vi "MegaAwesome_9_26_12b_JW.vi"() -> ()   [LabVIEW 2011]
uses:
  data/MegaAwesome_States.ctl
  <vilib>/Utility/inputDevices.llb/keyboardAcquire.vi
  <vilib>/Utility/file.llb/Read From Spreadsheet File (string).vi
  <vilib>/Utility/file.llb/Write To Spreadsheet File (string).vi
panel:
  out "Image Center X":i32
  in  "Disable Flag":bool
  out "Index":string
  in  "Slider Min":dbl=5.0
  in  "Slider Max":dbl=5.0
  out "Opj X Axis":string
  out "X Axis Display Type":string
  in  "Index-Sat":dbl=5.0
  in  "Index-Lin":dbl=5.0
  in  "IndexLog-Lin":dbl=5.0
  in  "IndexLog-Sat":dbl=5.0 caption="Num Pts"
  out "Lin Id-Log Used":dbl[](array[numeric])
  out "Lin-Vg Array-Log Used":dbl[](array[numeric])
  in  "New: Comments":string
  out "Save Array":string[][](array[string])
  out "Folder Index":i32 caption="Length"
  out "Sat Id-Used":dbl[](array[numeric])
  out "Sat Vg Array-Used":dbl[](array[numeric])
  out "Vg Array-Log-Used":dbl[](array[numeric])
  out "Sat Id-Log-Used":dbl[](array[numeric])
  out "Lin Id-Used":dbl[](array[numeric])
  out "Lin-Vg Array-Used":dbl[](array[numeric])
  out "Lin Vd":dbl
  out "Recorded Prop":T1
  out "Current State":T2
  in  "Main Tab Control":T3(tab)
  in  "Transfer File":path
  out "Transfer Folder":path
  in  "1) Transport":bool caption="2) Transport"
  in  "Image Analysis":bool caption="1) Image Analysis"
  in  "Transport\nFolder":path caption="Transport Folder"
  out "Transport\nFile":path=path "D:/UserData/Desktop/Jeremy/WFU/Research/Programs/VI mods/Image Not Found.png" caption="Transport File"
  in  "Image Folder":path
  out "Image File":path=path "D:/UserData/Desktop/Jeremy/WFU/Research/Programs/VI mods/Image Not Found.png"
  out "Fabrication Prop":T4
  out "Distances":dbl[](array[numeric])
  in  "Zoom":i16(slide)=-3 scale=-5.0..5.0
  in  "Magnification":u16(ring) items=["5x", "10x", "20x", "50x", "80x"]
  in  "Undo Button":bool
  in  "Remove Button":bool
  in  "Transfer Plots":T5(tab)=enum."Saturation"
  in  "Lin-Trans Slider":dbl(slide) step=1.0 scale=-2.0..2.0 scale format="%#_1p"
  out "Sqrt-Lin":cluster{dbl[], dbl[]}[](graph)
  in  "Sat-Trans Slider":dbl(slide) step=1.0 scale=-2.0..2.0 scale format="%#_1p"
  out "Sqrt-Sat":cluster{dbl[], dbl[]}[](graph)
  out "Raw- Lin":cluster{dbl[], dbl[]}[](graph)
  out "Raw- Sat":cluster{dbl[], dbl[]}[](graph)
  in  "Log Plots":enum32{"Linear", "Saturation", "Transport"}(tab)=enum."Saturation"
  in  "Lin-Log Slider":dbl(slide) step=1.0 scale=-2.0..2.0 scale format="%#_1p"
  out "Lin-Log":cluster{dbl[], dbl[]}[](graph)
  in  "Sat-Log Slider":dbl(slide) step=1.0 scale=-2.0..2.0 scale format="%#_1p"
  out "Sat-Log":cluster{dbl[], dbl[]}[](graph)
  out "Transport":cluster{ext[], ext[]}[](graph)
  out "Transport Name:":string
  in  "Manual Controls":T6
  in  "File Controls":T7
  out "Date Recorded":string="Date Recorded" caption="Measured"
  out "Data Name:":string
  out "Image Name":string
  out "Date Created":string caption="Fabricated"
  in  "Comments:":string
  out "Rec: Length":dbl caption="Length" format="%#_3g"
  out "Rec: Width":dbl caption="Width" format="%#_4g"
  out "Rec: Dielectric (d)":dbl caption="Dielectric (d)" format="%#_3g"
  in  "New: Dielectric":dbl
  in  "New: Length":dbl
  in  "New: Width":dbl
  out "Rec: Temp":dbl caption="Sample Temp" format="%.1f"
  in  "New: Temp":dbl format="%.1f"
  out "Image Out":T8(plugin-control)
  in  "Num Pts":dbl=5.0
  in  "Num Pts Log":dbl=5.0 caption="Num Pts"
  out "Recorded Values Cluster":T9
  out "Calculated Values Cluster":T9 caption="Recorded Values Cluster"
  out "Re-Calculated Values Cluster":T9 caption="Recorded Values Cluster"
  in  "Independant Variable:":string(combo)="Length (um):"
  out "Image Preview":T8(plugin-control)
  out "Total Width":dbl
  in  "Index Array":u16(ring) caption="Index" items=["1A", "1A", "1A", "1A", "1A", "1A", "1A", "1A", "1A", "1A", "1A", "1A", "1A", "1A", "1A", "1A", "1A", "1A", "1A", "1A", "1A", "1A", "1A", "1A", "1A", "1A", "1A", "1A", "1A", "1A", "1A", "1A", "1A", "1A", "1A", "1A", "1A"]
  in  "Room Temp":dbl=294.0 caption="Room Temp (K)"
  out "No Image\n File":path=path "\\\\acad1\\physics/Jurchescu-group/JW-PD/Mega Awesome/Image Not Found.png" caption="No Image File"
  out "Origin Project File":path=path "\\\\acad1\\physics/Jurchescu-group/JW-PD/Group Library/Origin Project Files/DeviceData_8_10_12a_JW.opj"
  out "No Transport\n File":path=path "\\\\acad1\\physics/Jurchescu-group/JW-PD/Mega Awesome/No Transport File.txt" caption="No Transport File"
  in  "Transport Style Controls":T10={"Transport Line Size"=1, "Transport Line Color"=16772608} {"Transport Line Size" items=["Extra Small", "Small", "Medium", "Large", "Extra Large"]}
  out "Application Directory":path
  # "1)  Select the Transfer File that you would like to analyze:"
  # "Transfer Location"
  # "2) What else would you like to view during your analysis?"
  # "Transport Location"
  # "Image Location"
  # "Recorded"
  # "Calculated"
  # "Re-Calculated"
  # "Manual"
  # "um"
  # "Slider\nDoesn't\nWork"
  # "V"
  # "V"
  # "Slider\nDoesn't\nWork"
  # "V"
  # "Default File Choices"
  # "Default Analysis Values"
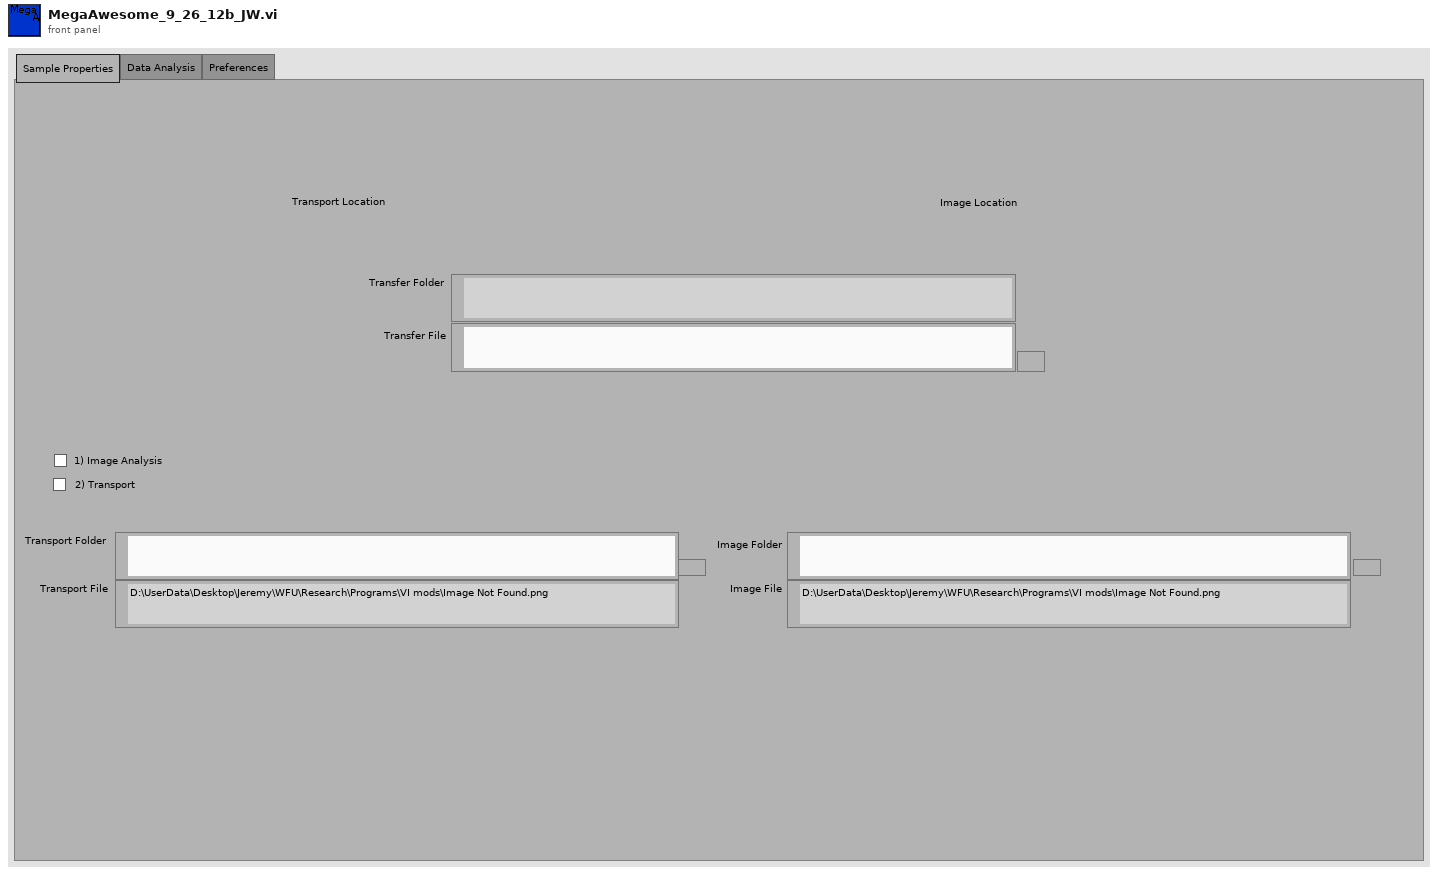
[diagram p1: front panel]
types:
  T1 = cluster{"Date Recorded":string, "Index":string, "Length":dbl, "Width":dbl, "Sample Temp":dbl}
  T2 = typedef "MegaAwesome_States.ctl" = enum16{"Init", "File Missing", "No Event", "Read Data", "Calculated Values", "Re-Calculated Values", "Next File", "Previous File", "Discard File", "Save", "Save Lines", "Export", "Exit"}
  T3 = enum32{"Sample Properties", "Data Analysis", "Preferences"}
  T4 = cluster{"Date Created":string, "Material":string, "Solvent":string, "Concentration":dbl, "Method":string, "Dielectric (nm)":dbl, "Treatment":string, "Comments":string}
  T5 = enum32{"Linear", "Saturation", "Raw-Linear", "Raw-Saturation"}
  T6 = cluster{"Manual-Temp":bool, "Manual-Width":bool, "Manuel-Length":bool, "Manuel-Dielectric":bool, "Manual Comments":bool}
  T7 = cluster{"Previous File":bool, "Discard ":bool, "Save Lines":bool, "Close":bool, "Next File ":bool, "Save":bool, "Save Next":bool, "Export":bool}
  T8 = typedef "IMAQ Image.ctl" = refnum<image>
  T9 = cluster{"Mobility-Sat":dbl, "Moblitity-Lin":dbl, "On/Off":dbl, "Off Current":dbl, "Vt-Sat":dbl, "STS":dbl, "Trap Density-VT":dbl, "Trap Density-STS":dbl}
  T10 = cluster{"Transport Line Size":u16, "Transport Line Color":u32}
  T11 = typedef "LVBoundsTypeDef.ctl" = cluster{"Width":u32, "Height":u32}
  T12 = cluster{"Global Rectangle":i32[], "Contours":cluster{"Contour Type":u32, "ROI Type":u32, "Points":i32[]}[]}
  T13 = cluster{"Contour Type":u32, "ROI Type":u32, "Points":i32[]}[]
  T14 = cluster{i32[], cluster{"Contour Type":u32, "ROI Type":u32, "Points":i32[]}[]}
  T15 = enum16{"0", "1", "2", "3", "4", "5", "6", "7", "8", "9", "A", "B", "C", "D", "E", "F", "G", "H", "I", "J", "K", "L", "M", "N", "O", "P", "Q", "R", "S", "T", "U", "V", "W", "X", "Y", "Z", "F1", "F2", "F3", "F4", "F5", "F6", "F7", "F8", "F9", "F10", "F11", "F12", "F13", "F14", "F15", "ADD", "BACK", "BACKSLASH", "CAPITAL", "COMMA", "DECIMAL", "DELETE", "DIVIDE", "DOWN", "END", "EQUALS", "ESCAPE", "GRAVE (`)", "HOME", "INSERT", "LBRACKET", "LCONTROL", "LEFT", "L ALT", "LSHIFT", "LWIN", "MINUS", "MULTIPLY", "NEXT", "NUMLOCK", "NUMPAD_0", "NUMPAD_1", "NUMPAD_2", "NUMPAD_3", "NUMPAD_4", "NUMPAD_5", "NUMPAD_6", "NUMPAD_7", "NUMPAD_8", "NUMPAD_9", "PAUSE", "PERIOD", "PRIOR (PG UP)", "RBRACKET", "RCONTROL", "RETURN", "RIGHT", "R ALT", "RSHIFT", "RWIN", "SCROLL", "SEMICOLON", "SLASH", "SPACE", "SUBTRACT", "TAB", "UP", "ENTER (num pad)", "' (quote)"}[]
  T16 = enum16{"0", "1", "2", "3", "4", "5", "6", "7", "8", "9", "A", "B", "C", "D", "E", "F", "G", "H", "I", "J", "K", "L", "M", "N", "O", "P", "Q", "R", "S", "T", "U", "V", "W", "X", "Y", "Z", "F1", "F2", "F3", "F4", "F5", "F6", "F7", "F8", "F9", "F10", "F11", "F12", "F13", "F14", "F15", "ADD", "BACK", "BACKSLASH", "CAPITAL", "COMMA", "DECIMAL", "DELETE", "DIVIDE", "DOWN", "END", "EQUALS", "ESCAPE", "GRAVE (`)", "HOME", "INSERT", "LBRACKET", "LCONTROL", "LEFT", "L ALT", "LSHIFT", "LWIN", "MINUS", "MULTIPLY", "NEXT", "NUMLOCK", "NUMPAD_0", "NUMPAD_1", "NUMPAD_2", "NUMPAD_3", "NUMPAD_4", "NUMPAD_5", "NUMPAD_6", "NUMPAD_7", "NUMPAD_8", "NUMPAD_9", "PAUSE", "PERIOD", "PRIOR (PG UP)", "RBRACKET", "RCONTROL", "RETURN", "RIGHT", "R ALT", "RSHIFT", "RWIN", "SCROLL", "SEMICOLON", "SLASH", "SPACE", "SUBTRACT", "TAB", "UP", "ENTER (num pad)", "' (quote)"}
  T17 = typedef "ROI Descriptor" = cluster{"Global Rectangle":i32[], "Contours":cluster{"ID":enum32{"External", "Internal"}, "Type":u32, "Coordinates":i32[]}[]}
  T18 = cluster{string, sgl, bool, bool, bool, bool, bool, bool, i32}
  T19 = cluster{i32, cluster{string, sgl, bool, bool, bool, bool, bool, bool, i32}, i32, i32}
  T20 = cluster{"Contour Type":u32, "ROI Type":u32, "Points":i32[]}
  T21 = cluster{"Points[0]":i32, "Points[1]":i32, "Points[2]":i32, "Points[3]":i32, "Points[4]":i32, "Points[5]":i32, "Points[6]":i32, "Points[7]":i32, "Points[8]":i32}
  T22 = cluster{"[0]":cluster{dbl[], dbl[]}, "[1]":cluster{dbl[], dbl[]}, "[2]":cluster{dbl[], dbl[]}, "[3]":cluster{dbl[], dbl[]}, "[4]":cluster{dbl[], dbl[]}, "[5]":cluster{dbl[], dbl[]}, "[6]":cluster{dbl[], dbl[]}, "[7]":cluster{dbl[], dbl[]}, "[8]":cluster{dbl[], dbl[]}}
  T23 = cluster{"Sat Vg Used":dbl[], "Sat Sqrt(Id) Used ":dbl[], "Lin Vg Used":dbl[], "Lin Sqrt(Id) Used":dbl[], "Index-Lin":dbl, "Index-Sat":dbl}
  T24 = cluster{"Raw Sat":cluster{dbl[], dbl[]}[], "Sqrt Sat":cluster{dbl[], dbl[]}[], "Log Sat":cluster{dbl[], dbl[]}[], "Raw Lin":cluster{dbl[], dbl[]}[], "Sqrt Lin":cluster{dbl[], dbl[]}[], "Log Lin":cluster{dbl[], dbl[]}[]}
  T25 = cluster{"Mobility-Sat":dbl, "Vt-Sat":dbl, "Mobility-Lin":dbl, "Vt-Lin":dbl, "Off I-Sat":dbl, "On/Off I-Sat":dbl}
  T26 = cluster{"Sat Vg Used":dbl[], "Sat Log(Id) Used":dbl[], "Lin Vg Used":dbl[], "Lin Log(Id) Used":dbl[], "STS Index-Sat":dbl, "STS Index-Lin":dbl}
  T27 = cluster{"Independant  Variable Indicator":string, "Parameter String Indicator":string}
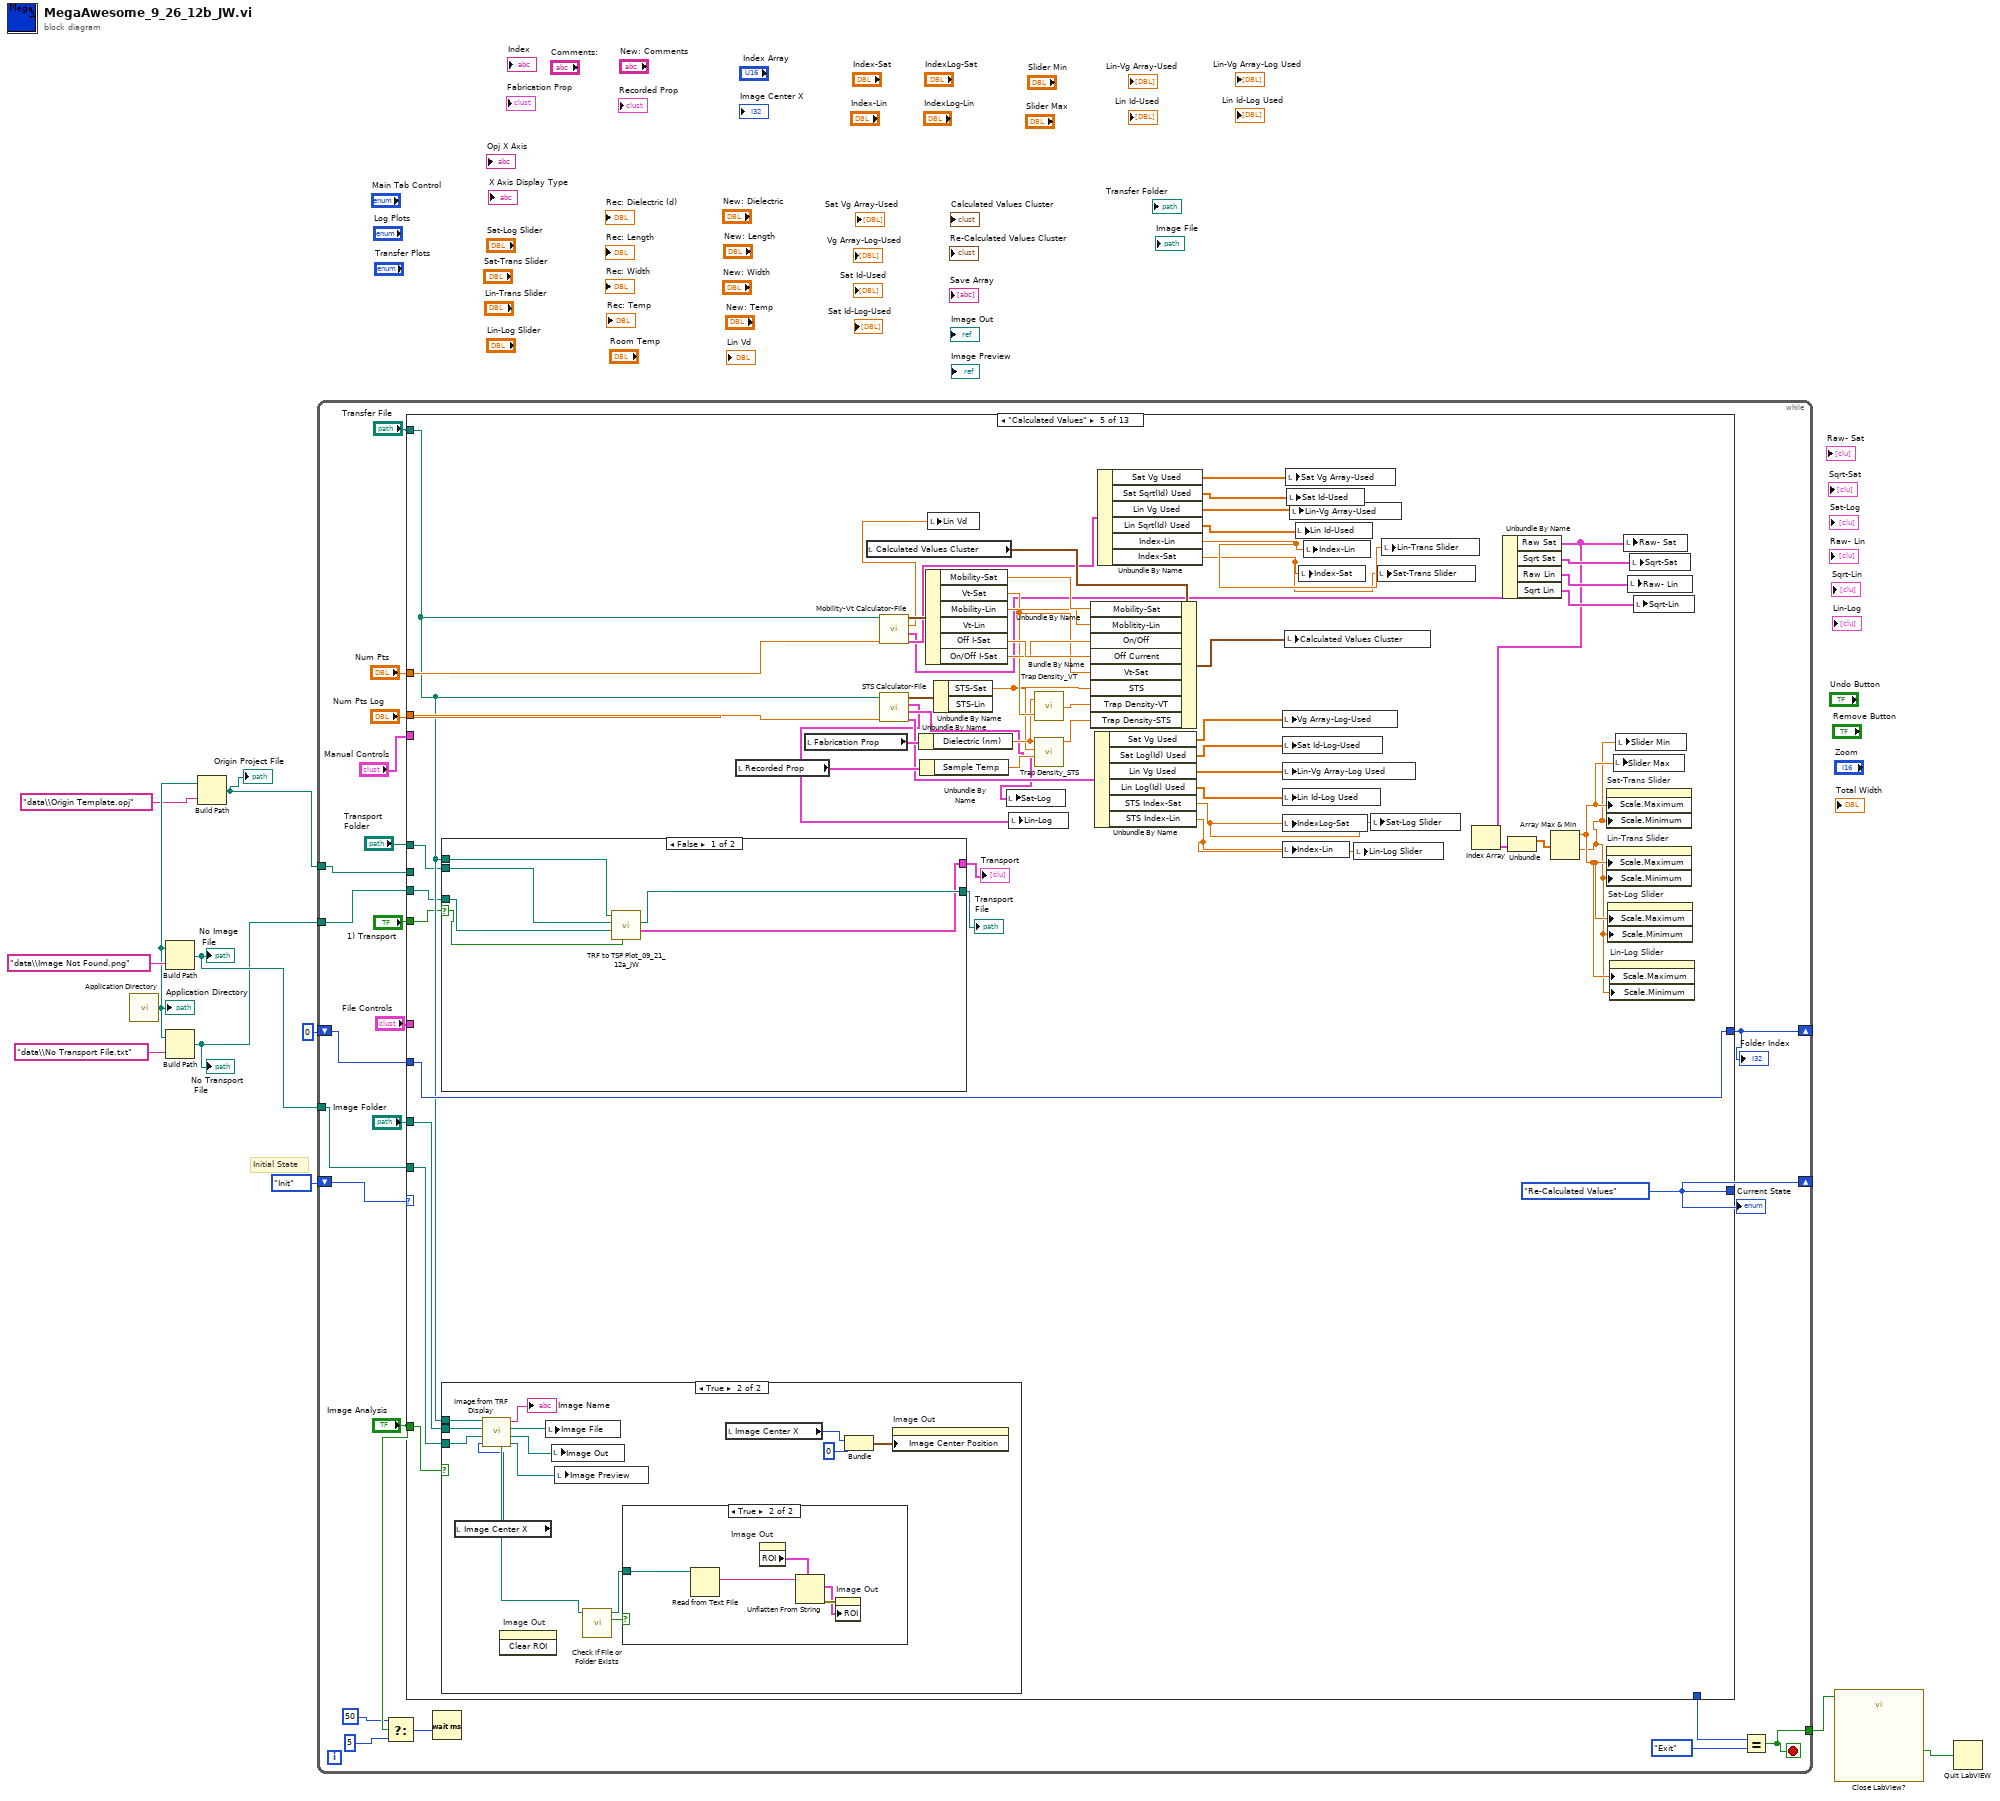
[diagram p0: block diagram]
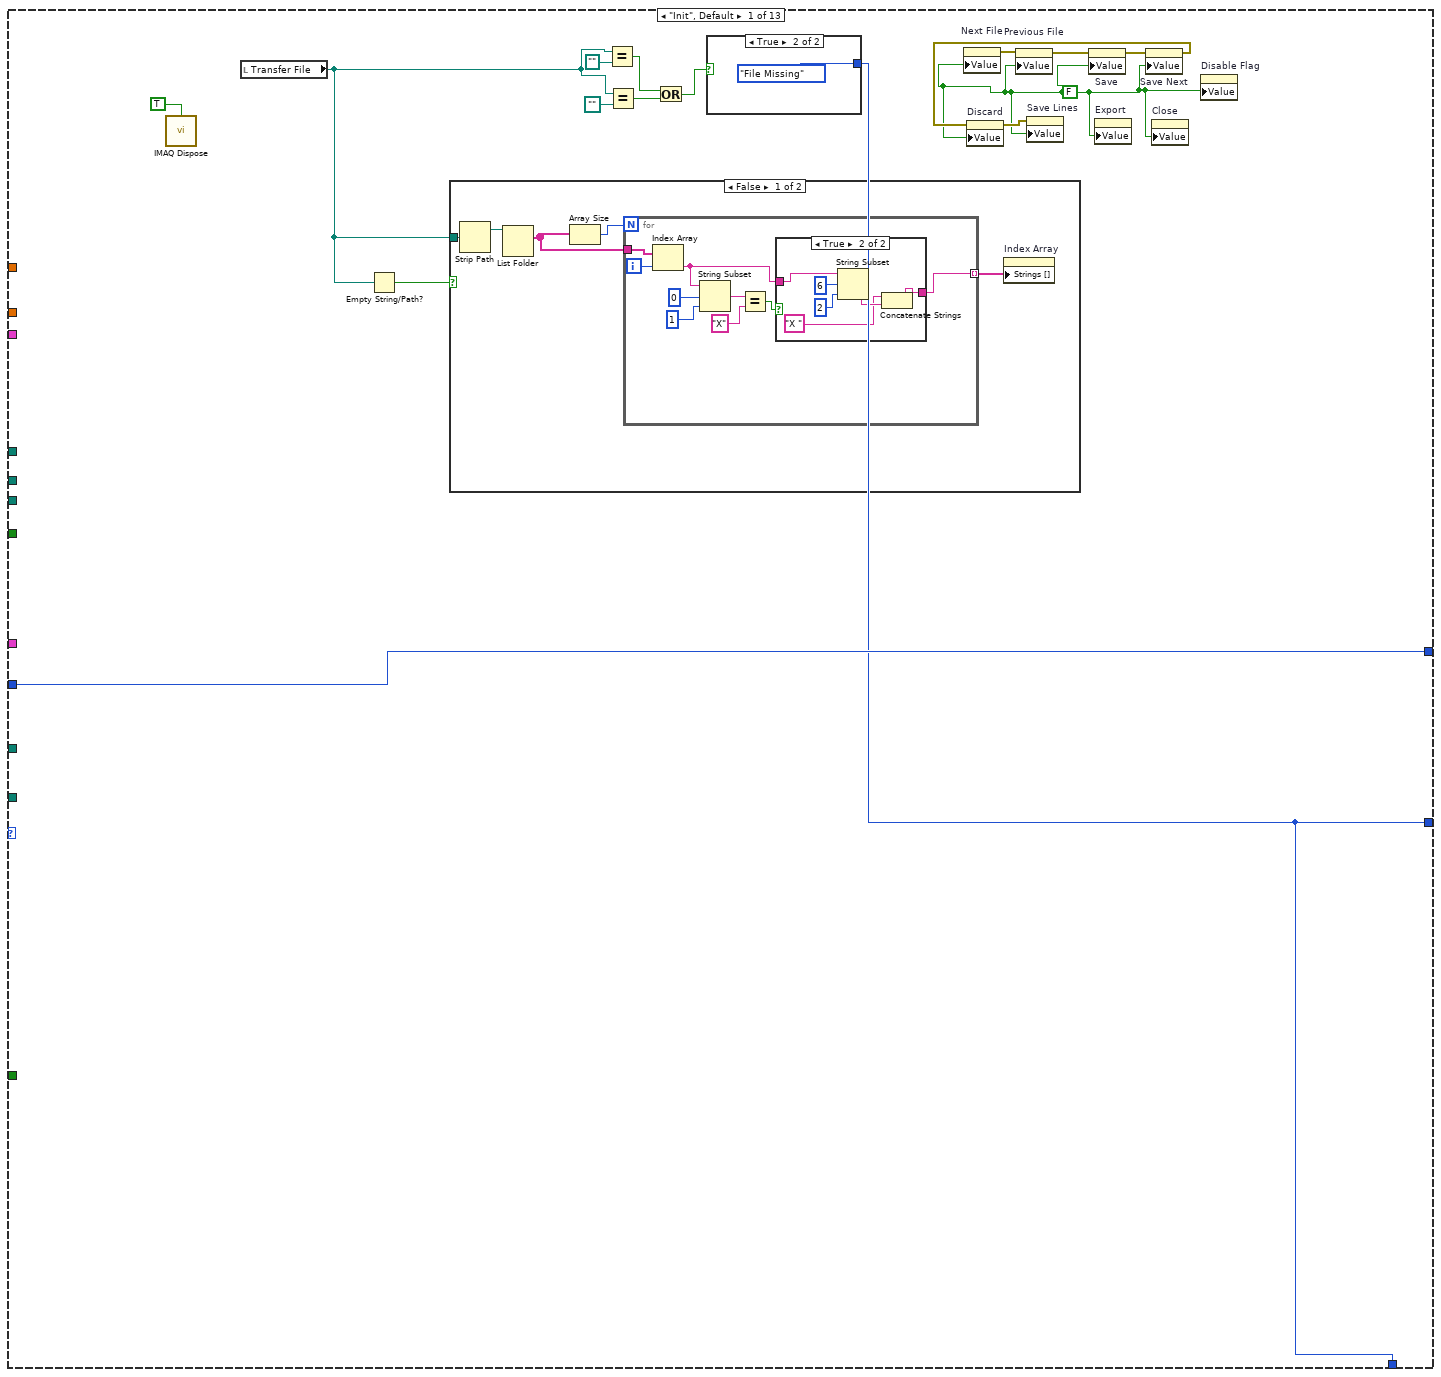
[diagram p2: hidden frame]
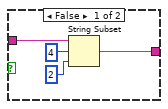
[diagram p3: hidden frame]
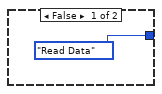
[diagram p5: hidden frame]
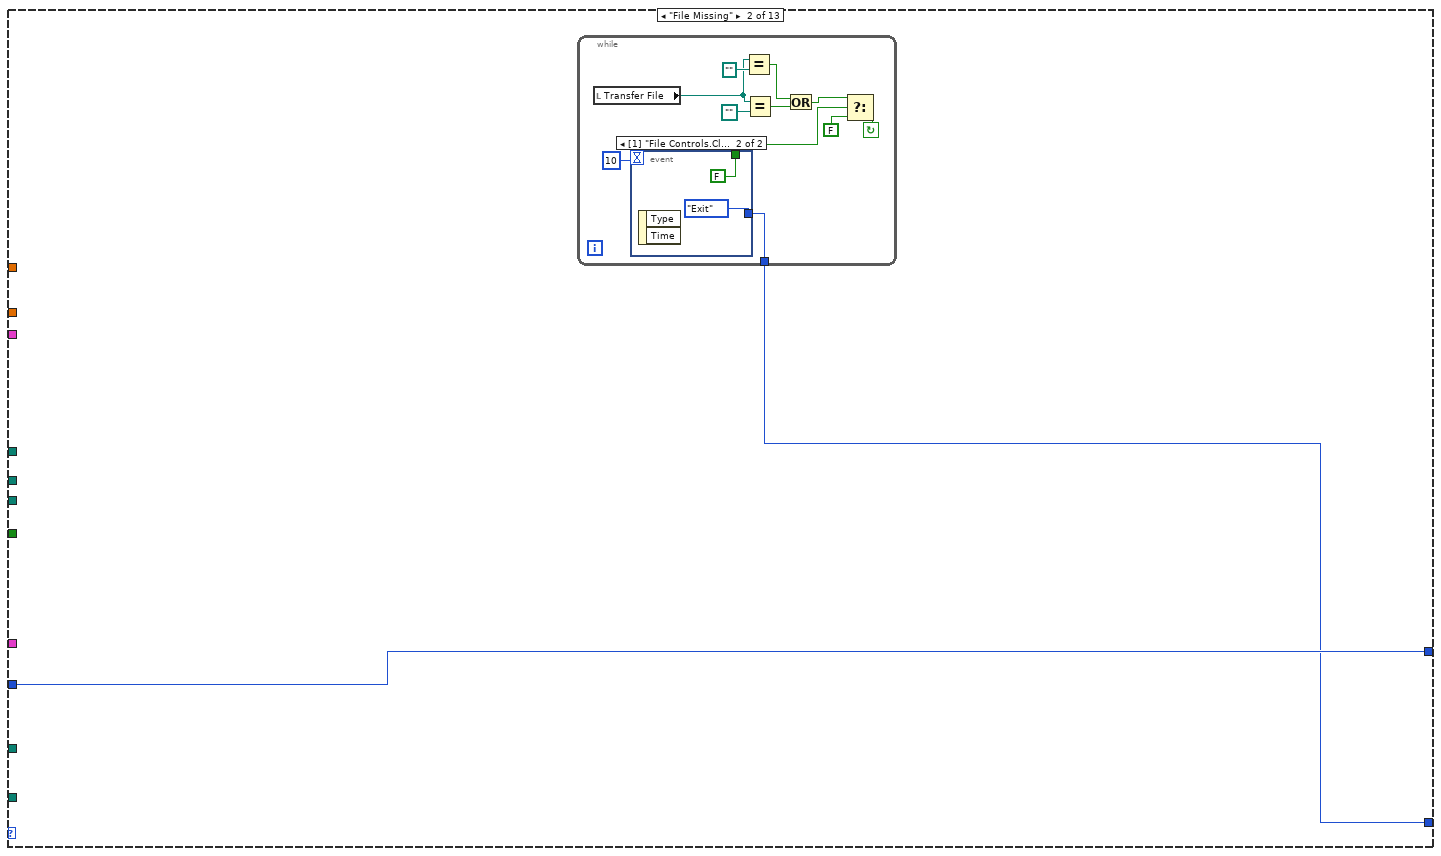
[diagram p6: hidden frame]
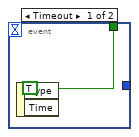
[diagram p7: hidden frame]
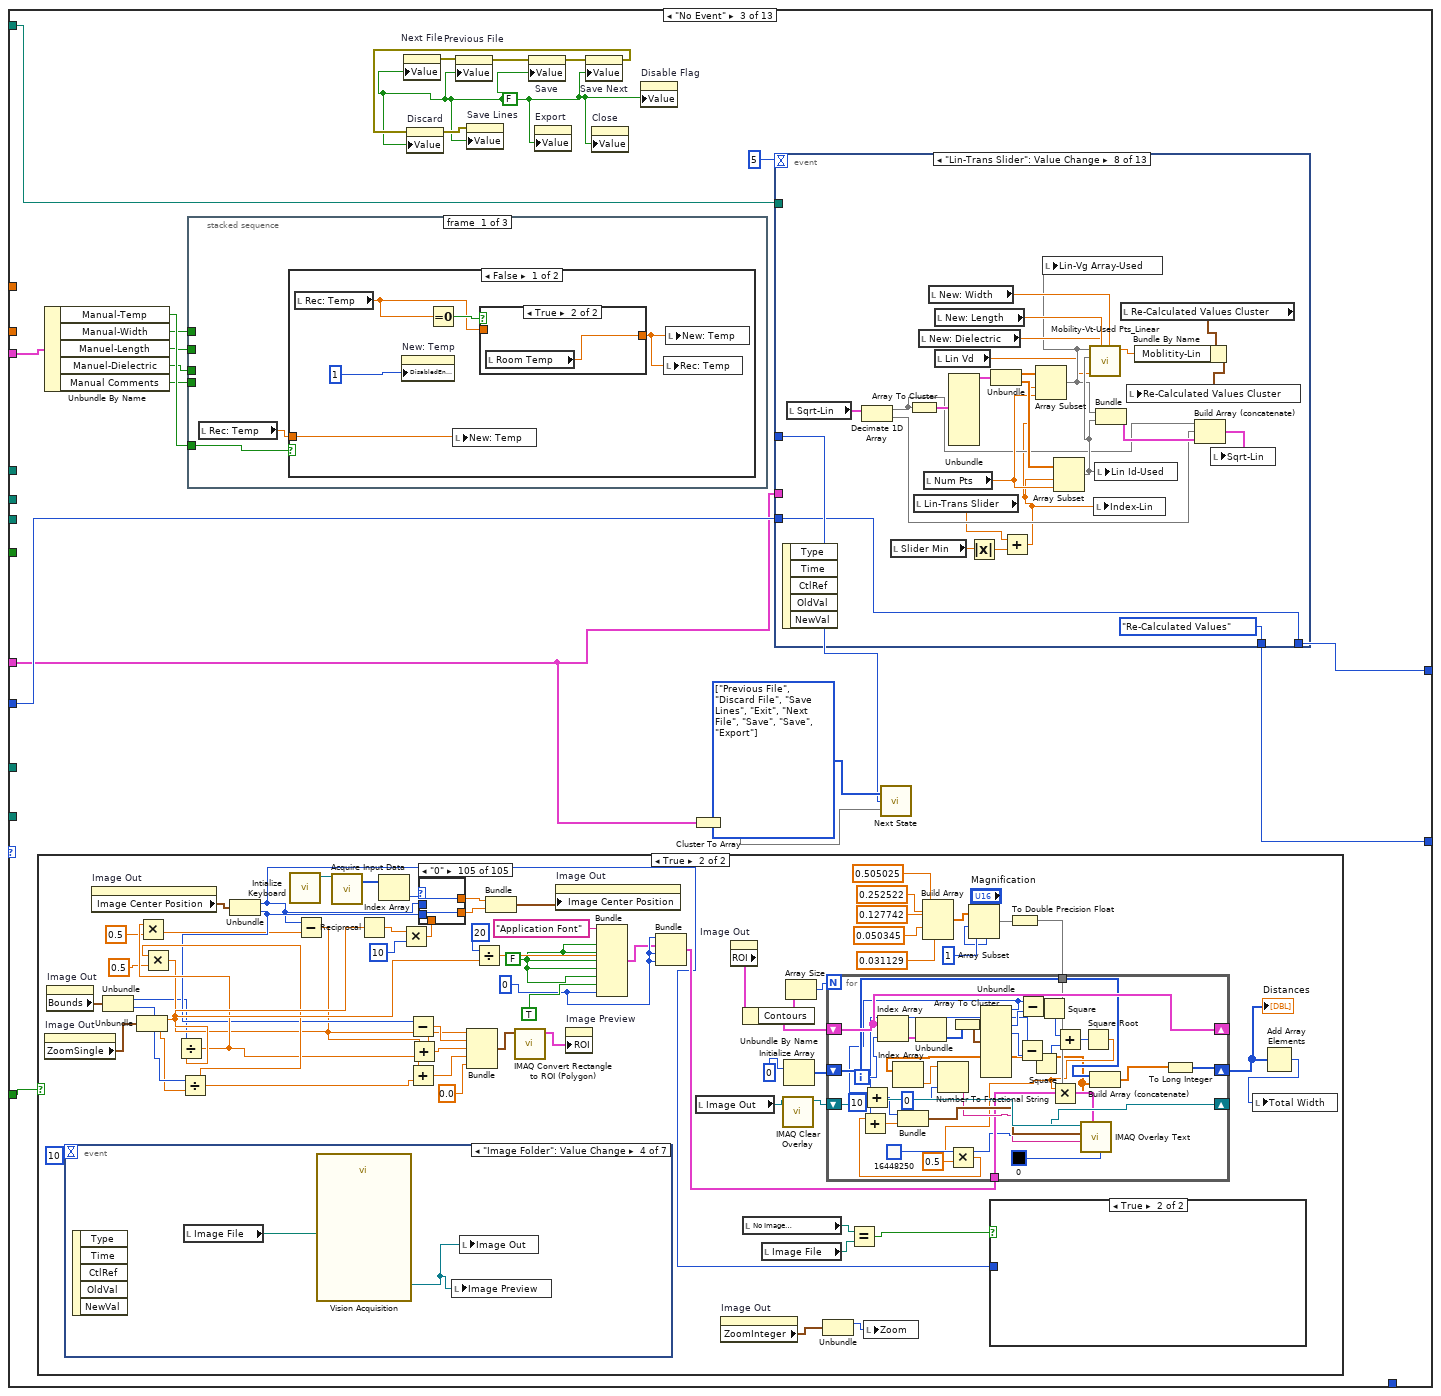
[diagram p8: hidden frame]
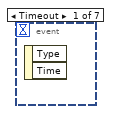
[diagram p10: hidden frame]
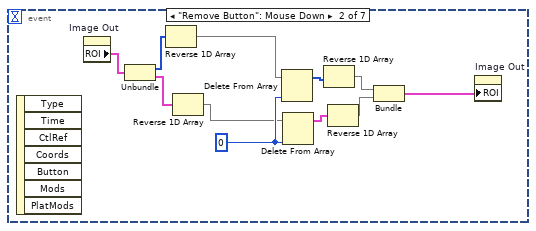
[diagram p11: hidden frame]
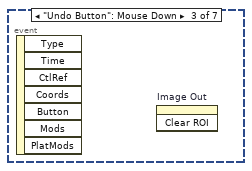
[diagram p12: hidden frame]
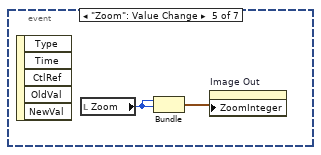
[diagram p13: hidden frame]
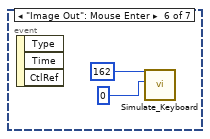
[diagram p14: hidden frame]
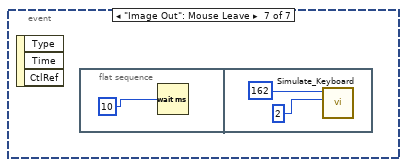
[diagram p15: hidden frame]
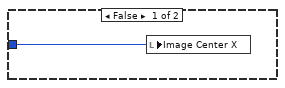
[diagram p16: hidden frame]
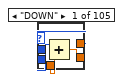
[diagram p17: hidden frame]
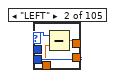
[diagram p18: hidden frame]
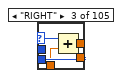
[diagram p19: hidden frame]
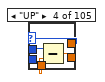
[diagram p20: hidden frame]
diagram:
  # "Initial State"
  n1 = call <vilib>:"Application Directory.vi"() -> ("Application Directory"=w4:path)
  "Application Directory" <- w4
  n2 = Build Path(base path=w4, name or relative path="data\\Image Not Found.png") -> (appended path=w7:path)
  "No Image\n File" <- w7
  n3 = Build Path(base path=w4, name or relative path="data\\No Transport File.txt") -> (appended path=w6:path)
  "No Transport\n File" <- w6
  n4 = Build Path(base path=w4, name or relative path="data\\Origin Template.opj") -> (appended path=w5:path)
  "Origin Project File" <- w5
  n5 = while {
    shift-right: [w15] -> _
    shift-left: MegaAwesome_States."Init" -> [w13]
    shift-right: [w27] -> _
    shift-left: 0 -> [w28]
    tunnel: w7 -> [w19]
    tunnel: w6 -> [w17]
    tunnel: w5 -> [w16]
    tunnel: [w14] -> w2
    stop <- w14 stop-if-true
    n6 = Select(t=50, s="Image Analysis", f=5) -> (s? t:f=w21:i32)
    n7 = case shown="\"Calculated Values\"" w13 {
      tunnel: [w34 w76 w104 MegaAwesome_States."Calculated Values" MegaAwesome_States."Re-Calculated Values" MegaAwesome_States."No Event" MegaAwesome_States."Read Data" MegaAwesome_States."Read Data" MegaAwesome_States."Init" w840 w1361 MegaAwesome_States."No Event" MegaAwesome_States."Exit"] -> w15
      tunnel: "Transfer File" -> [_ _ w94 w614 w662 _ w781 w792 w810 w845 _ _ _]
      tunnel: "Num Pts" -> [_ _ _ _ w685 _ _ _ _ _ _ _ _]
      tunnel: "Num Pts Log" -> [_ _ _ _ w684 _ _ _ _ _ _ _ _]
      tunnel: "Image Folder" -> [_ _ _ _ w681 _ _ _ _ _ _ w1372 _]
      tunnel: w19 -> [_ _ _ _ w680 _ _ _ _ _ _ _ _]
      tunnel: [w44 w77 w95 w619 w679 w741 w767 w790 w805 w846 w1362 w1382 w1388] -> w27
      tunnel: w28 -> [w44 w77 w96 w617 w679 w741 w768 w791 _ w846 w1362 w1382 w1388]
      tunnel: "Manual Controls" -> [_ _ w106 _ _ _ _ _ _ w844 _ _ _]
      tunnel: "File Controls" -> [_ _ w92 _ _ _ _ _ _ w839 _ _ _]
      tunnel: "1) Transport" -> [_ _ _ _ w653 _ _ _ _ _ _ _ _]
      tunnel: "Image Analysis" -> [_ _ w97 _ w652 _ _ _ _ _ _ _ _]
      tunnel: "Transport\nFolder" -> [_ _ _ _ w651 _ _ _ _ _ _ _ _]
      tunnel: w17 -> [_ _ _ _ w650 _ _ _ _ _ _ _ _]
      tunnel: w16 -> [_ _ _ _ _ _ _ _ _ _ _ _ w1387]
      tunnel: [w34 _ _ _ _ _ _ _ _ _ w1360 _ _] -> w12
      frame "Init", Default {
        w35 = FALSE
        n8 = call "IMAQ Dispose"("All Images? (No)"=TRUE) -> ()  [unwired: 5 in, 1 out]
        n9 = local read "Transfer File"() -> (w42:path)
        n10 = Empty String/Path?(string/path=w42) -> (empty?=w43:bool)
        n11 = case shown="False" w43 {
          tunnel: w42 -> [w51 _]
          frame False {
            n12 = Strip Path(path=w51) -> (stripped path=w53:path)  [unwired: 1 out]
            n13 = List Folder(path=w53) -> (filenames=w52:string[])  [unwired: 3 in, 3 out]
            n14 = Array Size(array=w52) -> (size(s)=w54:i32)
            n15 = for {
              N: w54 -> [_]
              tunnel: w52 -> [w63]
              tunnel: [w61] -> w50 mode=indexing
              i -> [w62]
              n16 = Index Array(array=w63, index=w62) -> (element=w60:string)
              n17 = String Subset(string=w60, offset (0)=0, length (rest)=1) -> (substring=w57:string)
              n18 = Equal?(x=w57, y="X") -> (x = y?=w56:bool)
              n19 = case shown="True" w56 {
                tunnel: w60 -> [w67 w71]
                tunnel: [w64 w70] -> w61
                frame False {
                  n20 = String Subset(string=w67, offset (0)=4, length (rest)=2) -> (substring=w64:string)
                }
                frame True {
                  n21 = String Subset(string=w71, offset (0)=6, length (rest)=2) -> (substring=w69:string)
                  n22 = Concatenate Strings("X ", w69) -> (w70:string)
                }
              }
            }
            n23 = property on="Index Array" class="Ring (strict)"("Strings []"=w50) -> ()  [unwired: 2 in, 2 out]
          }
          frame True {
          }
        }
        n24 = Equal?(x=w42, y=path "") -> (x = y?=w47:bool)
        n25 = Equal?(x=w42, y=path "") -> (x = y?=w46:bool)
        n26 = Or(x=w47, y=w46) -> (x .or. y?=w49:bool)
        n27 = case shown="True" w49 {
          tunnel: [MegaAwesome_States."Read Data" MegaAwesome_States."File Missing"] -> w34
          frame False {
          }
          frame True {
          }
        }
        n28 = property on="Next File" class="Bool (strict)"("Value"=w35) -> (error out=w40:errorcluster)  [unwired: 2 in, 1 out]
        n29 = property on="Previous File" class="Bool (strict)"(error in=w40, "Value"=w35) -> (error out=w39:errorcluster)  [unwired: 1 in, 1 out]
        n30 = property on="Save" class="Bool (strict)"(error in=w39, "Value"=w35) -> (error out=w38:errorcluster)  [unwired: 1 in, 1 out]
        n31 = property on="Export" class="Bool (strict)"("Value"=w35) -> ()  [unwired: 2 in, 2 out]
        n32 = property on="Save Next" class="Bool (strict)"(error in=w38, "Value"=w35) -> (error out=w37:errorcluster)  [unwired: 1 in, 1 out]
        n33 = property on="Discard" class="Bool (strict)"(error in=w37, "Value"=w35) -> (error out=w36:errorcluster)  [unwired: 1 in, 1 out]
        n34 = property on="Save Lines" class="Bool (strict)"(error in=w36, "Value"=w35) -> ()  [unwired: 1 in, 2 out]
        n35 = property on="Close" class="Bool (strict)"("Value"=w35) -> ()  [unwired: 2 in, 2 out]
        n36 = property on="Disable Flag" class="Bool (strict)"("Value"=w35) -> ()  [unwired: 2 in, 2 out]
      }
      frame "File Missing" {
        n37 = while {
          tunnel: [w83] -> w76
          stop <- w79 continue-if-true
          n38 = local read "Transfer File"() -> (w84:path)
          n39 = event shown="[1] \"File Controls.Close\": Value Change" {
            selector: _ -> [_ _]
            dyn-events: _ -> [_ _]
            timeout: 10 -> [_ _]
            tunnel: [_ MegaAwesome_States."Exit"] -> w83
            tunnel: [TRUE FALSE] -> w82
            event Timeout {
              n40 = event-data() -> ()  [unwired: 1 in, 2 out]
            }
            event "File Controls.Close": Value Change {
              n41 = event-data() -> ()  [unwired: 1 in, 2 out]
            }
          }
          n42 = Equal?(x=w84, y=path "") -> (x = y?=w86:bool)
          n43 = Equal?(x=w84, y=path "") -> (x = y?=w87:bool)
          n44 = Or(x=w86, y=w87) -> (x .or. y?=w81:bool)
          n45 = Select(t=w81, s=w82, f=FALSE) -> (s? t:f=w79:bool)
        }
      }
      frame "No Event" {
        w93 = FALSE
        w113 = T2[] [enum."Previous File", enum."Discard File", enum."Save Lines", enum."Exit", enum."Next File", enum."Save", enum."Save", enum."Export"] items=["Init", "File Missing", "No Event", "Read Data", "Calculated Values", "Re-Calculated Values", "Next File", "Previous File", "Discard File", "Save", "Save Lines", "Export", "Exit"]
        n46 = case shown="True" w97 {
          frame False {
          }
          frame True {
            w169 = FALSE
            w171 = 0
            n47 = property on="Image Out" class="ImageControl"() -> ("ZoomSingle"=w155:cluster{"X":sgl, "Y":sgl})  [unwired: 2 in, 2 out]
            n48 = property on="Image Out" class="ImageControl"() -> ("Bounds"=w154:T11)  [unwired: 2 in, 2 out]
            n49 = event shown="[3] \" Image Folder\": Value Change" {
              selector: _ -> [_ _ _ _ _ _ _]
              dyn-events: _ -> [_ _ _ _ _ _ _]
              timeout: 10 -> [_ _ _ _ _ _ _]
              event Timeout {
                n50 = event-data() -> ()  [unwired: 1 in, 2 out]
              }
              event "Remove Button": Mouse Down {
                w188 = 0
                n51 = event-data() -> ()  [unwired: 1 in, 7 out]
                n52 = property on="Image Out" class="ImageControl"() -> ("ROI"=w178:T12)  [unwired: 2 in, 2 out]
                n53 = Unbundle(w178) -> ("Global Rectangle"=w187:i32[], "Contours"=w185:T13)
                n54 = Reverse 1D Array(array=w187) -> (reversed array=w186:i32[])
                n55 = Reverse 1D Array(array=w185) -> (reversed array=w184:T13)
                n56 = Delete From Array(array=w186, index=w188) -> (array with subset deleted=w183:i32[])  [unwired: 1 in, 1 out]
                n57 = Delete From Array(array=w184, index=w188) -> (array with subset deleted=w182:T13)  [unwired: 1 in, 1 out]
                n58 = Reverse 1D Array(array=w183) -> (reversed array=w181:i32[])
                n59 = Reverse 1D Array(array=w182) -> (reversed array=w180:T13)
                n60 = Bundle(w181, w180) -> (w179:T14)  [unwired: 1 in]
                n61 = property on="Image Out" class="ImageControl"("ROI"=w179) -> ()  [unwired: 2 in, 2 out]
              }
              event "Undo Button": Mouse Down {
                n62 = event-data() -> ()  [unwired: 1 in, 7 out]
                n63 = invoke on="Image Out" class="ImageControl" method="Clear ROI"() -> ()  [unwired: 3 in, 3 out]
              }
              event "Image Folder": Value Change {
                n64 = event-data() -> ()  [unwired: 1 in, 5 out]
                n65 = local read "Image File"() -> (w190:path)
                n66 = call "Vision Acquisition"("Image Path"=w190) -> ("Image Out"=w189:T8)  [unwired: 25 in, 1 out]
                n67 = local write "Image Preview"(w189) -> ()
                n68 = local write "Image Out"(w189) -> ()
              }
              event "Zoom": Value Change {
                n69 = event-data() -> ()  [unwired: 1 in, 5 out]
                n70 = local read "Zoom"() -> (w191:i16)
                n71 = Bundle("Zoom"=w191, "Zoom"=w191) -> (w192:cluster{"Zoom":i16, "Zoom":i16})  [unwired: 1 in]
                n72 = property on="Image Out" class="ImageControl"("ZoomInteger"=w192) -> ()  [unwired: 2 in, 2 out]
              }
              event "Image Out": Mouse Enter {
                n73 = event-data() -> ()  [unwired: 1 in, 3 out]
                n74 = call "Simulate_Keyboard.vi"("Action"=0, "Virtual Key"=162) -> ()  [unwired: 7 in, 1 out]
              }
              event "Image Out": Mouse Leave {
                n75 = event-data() -> ()  [unwired: 1 in, 3 out]
                n76 = flat-sequence {
                  frame #0 {
                    n77 = Wait (ms)(milliseconds to wait=10) -> ()  [unwired: 1 out]
                  }
                  frame #1 {
                    n78 = call "Simulate_Keyboard.vi"("Action"=2, "Virtual Key"=162) -> ()  [unwired: 7 in, 1 out]
                  }
                }
              }
            }
            n79 = property on="Image Out" class="ImageControl"() -> ("Image Center Position"=w148:cluster{"X":u32, "Y":u32})  [unwired: 2 in, 2 out]
            n80 = Unbundle(w154) -> ("Width"=w157:u32, "Height"=w158:u32)
            n81 = Unbundle(w155) -> ("X"=w175:sgl, "Y"=w156:sgl)
            n82 = Divide(x=w157, y=w175) -> (x/y=w166:sgl)
            n83 = Multiply(x=w166, y=0.5) -> (x*y=w161:dbl)
            n84 = Divide(x=w158, y=w156) -> (x/y=w167:sgl)
            n85 = Multiply(x=w167, y=0.5) -> (x*y=w162:dbl)
            n86 = Unbundle(w148) -> ("X"=w120:u32, "Y"=w165:u32)
            n87 = call <vilib>:"Intialize Keyboard.vi"() -> ("device ID"=w145:refnum<k1>)  [unwired: 10 in, 1 out]
            n88 = Subtract(x=w120, y=w161) -> (x-y=w163:dbl)
            n89 = call-poly <vilib>:"Acquire Input Data.vi"("device ID"=w145) -> ("keys pressed"=w146:T15)  [unwired: 16 in, 2 out]
            n90 = Reciprocal(x=w175) -> (1/x=w176:sgl)
            n91 = Index Array(array=w146) -> (element=w142:T16)  [unwired: 1 in]
            n92 = Multiply(x=w176, y=10) -> (x*y=w174:sgl)
            n93 = Subtract(x=w165, y=w162) -> (x-y=w164:dbl)
            n94 = Add(x=w164, y=w167) -> (x+y=w150:dbl)
            n95 = Add(x=w163, y=w166) -> (x+y=w149:dbl)
            n96 = case shown="\"0\"" w142 {
              tunnel: w120 -> [w234 w240 w244 w246 w250 w252 w254 w256 w258 w260 w262 w264 w266 w268 w270 w272 w274 w276 w278 w280 w282 w284 w286 w288 w290 w292 w294 w296 w298 w300 w302 w304 w306 w308 w310 w312 w314 w316 w318 w320 w322 w324 w326 w328 w330 w332 w334 w336 w338 w340 w342 w344 w346 w348 w350 w352 w354 w356 w358 w360 w362 w364 w366 w368 w370 w372 w374 w376 w378 w380 w382 w384 w386 w388 w390 w392 w394 w396 w398 w400 w402 w404 w406 w408 w410 w412 w414 w416 w418 w420 w422 w424 w426 w428 w430 w432 w434 w436 w438 w440 w442 w444 w446 w448 w450]
              tunnel: [w234 w239 w243 w246 w250 w252 w254 w256 w258 w260 w262 w264 w266 w268 w270 w272 w274 w276 w278 w280 w282 w284 w286 w288 w290 w292 w294 w296 w298 w300 w302 w304 w306 w308 w310 w312 w314 w316 w318 w320 w322 w324 w326 w328 w330 w332 w334 w336 w338 w340 w342 w344 w346 w348 w350 w352 w354 w356 w358 w360 w362 w364 w366 w368 w370 w372 w374 w376 w378 w380 w382 w384 w386 w388 w390 w392 w394 w396 w398 w400 w402 w404 w406 w408 w410 w412 w414 w416 w418 w420 w422 w424 w426 w428 w430 w432 w434 w436 w438 w440 w442 w444 w446 w448 w450] -> w143
              tunnel: w165 -> [w236 w238 w242 w248 w249 w251 w253 w255 w257 w259 w261 w263 w265 w267 w269 w271 w273 w275 w277 w279 w281 w283 w285 w287 w289 w291 w293 w295 w297 w299 w301 w303 w305 w307 w309 w311 w313 w315 w317 w319 w321 w323 w325 w327 w329 w331 w333 w335 w337 w339 w341 w343 w345 w347 w349 w351 w353 w355 w357 w359 w361 w363 w365 w367 w369 w371 w373 w375 w377 w379 w381 w383 w385 w387 w389 w391 w393 w395 w397 w399 w401 w403 w405 w407 w409 w411 w413 w415 w417 w419 w421 w423 w425 w427 w429 w431 w433 w435 w437 w439 w441 w443 w445 w447 w449]
              tunnel: [w235 w238 w242 w247 w249 w251 w253 w255 w257 w259 w261 w263 w265 w267 w269 w271 w273 w275 w277 w279 w281 w283 w285 w287 w289 w291 w293 w295 w297 w299 w301 w303 w305 w307 w309 w311 w313 w315 w317 w319 w321 w323 w325 w327 w329 w331 w333 w335 w337 w339 w341 w343 w345 w347 w349 w351 w353 w355 w357 w359 w361 w363 w365 w367 w369 w371 w373 w375 w377 w379 w381 w383 w385 w387 w389 w391 w393 w395 w397 w399 w401 w403 w405 w407 w409 w411 w413 w415 w417 w419 w421 w423 w425 w427 w429 w431 w433 w435 w437 w439 w441 w443 w445 w447 w449] -> w144
              tunnel: w174 -> [w233 w237 w241 w245 _ _ _ _ _ _ _ _ _ _ _ _ _ _ _ _ _ _ _ _ _ _ _ _ _ _ _ _ _ _ _ _ _ _ _ _ _ _ _ _ _ _ _ _ _ _ _ _ _ _ _ _ _ _ _ _ _ _ _ _ _ _ _ _ _ _ _ _ _ _ _ _ _ _ _ _ _ _ _ _ _ _ _ _ _ _ _ _ _ _ _ _ _ _ _ _ _ _ _ _ _]
              frame "DOWN" {
                n97 = Add(x=w236, y=w233) -> (x+y=w235:sgl)
              }
              frame "LEFT" {
                n98 = Subtract(x=w240, y=w237) -> (x-y=w239:sgl)
              }
              frame "RIGHT" {
                n99 = Add(x=w244, y=w241) -> (x+y=w243:sgl)
              }
              frame "UP" {
                n100 = Subtract(x=w248, y=w245) -> (x-y=w247:sgl)
              }
              frame "ENTER (num pad)" {
              }
              frame "' (quote)" {
              }
              frame "END" {
              }
              frame "EQUALS" {
              }
              frame "ESCAPE" {
              }
              frame "GRAVE (`)" {
              }
              frame "HOME" {
              }
              frame "INSERT" {
              }
              frame "LBRACKET" {
              }
              frame "LCONTROL" {
              }
              frame "L ALT" {
              }
              frame "LSHIFT" {
              }
              frame "LWIN" {
              }
              frame "MINUS" {
              }
              frame "MULTIPLY" {
              }
              frame "NEXT" {
              }
              frame "NUMLOCK" {
              }
              frame "NUMPAD_0" {
              }
              frame "NUMPAD_1" {
              }
              frame "NUMPAD_2" {
              }
              frame "NUMPAD_3" {
              }
              frame "NUMPAD_4" {
              }
              frame "NUMPAD_5" {
              }
              frame "NUMPAD_6" {
              }
              frame "NUMPAD_7" {
              }
              frame "NUMPAD_8" {
              }
              frame "NUMPAD_9" {
              }
              frame "PAUSE" {
              }
              frame "PERIOD" {
              }
              frame "PRIOR (PG UP)" {
              }
              frame "RBRACKET" {
              }
              frame "RCONTROL" {
              }
              frame "RETURN" {
              }
              frame "R ALT" {
              }
              frame "RSHIFT" {
              }
              frame "RWIN" {
              }
              frame "SCROLL" {
              }
              frame "SEMICOLON" {
              }
              frame "SLASH" {
              }
              frame "SPACE" {
              }
              frame "SUBTRACT" {
              }
              frame "TAB" {
              }
              frame "DIVIDE" {
              }
              frame "DELETE" {
              }
              frame "DECIMAL" {
              }
              frame "COMMA" {
              }
              frame "CAPITAL" {
              }
              frame "BACKSLASH" {
              }
              frame "BACK" {
              }
              frame "ADD" {
              }
              frame "F15" {
              }
              frame "F14" {
              }
              frame "F13" {
              }
              frame "F12" {
              }
              frame "F11" {
              }
              frame "F10" {
              }
              frame "F9" {
              }
              frame "F8" {
              }
              frame "F7" {
              }
              frame "F6" {
              }
              frame "F5" {
              }
              frame "F4" {
              }
              frame "F3" {
              }
              frame "F2" {
              }
              frame "F1" {
              }
              frame "Z" {
              }
              frame "Y" {
              }
              frame "X" {
              }
              frame "W" {
              }
              frame "V" {
              }
              frame "U" {
              }
              frame "T" {
              }
              frame "S" {
              }
              frame "R" {
              }
              frame "Q" {
              }
              frame "P" {
              }
              frame "O" {
              }
              frame "N" {
              }
              frame "M" {
              }
              frame "L" {
              }
              frame "K" {
              }
              frame "J" {
              }
              frame "I" {
              }
              frame "H" {
              }
              frame "G" {
              }
              frame "F" {
              }
              frame "E" {
              }
              frame "D" {
              }
              frame "C" {
              }
              frame "B" {
              }
              frame "A" {
              }
              frame "9" {
              }
              frame "8" {
              }
              frame "7" {
              }
              frame "6" {
              }
              frame "5" {
              }
              frame "4" {
              }
              frame "3" {
              }
              frame "2" {
              }
              frame "1" {
              }
              frame "0" {
              }
            }
            n101 = Bundle(w163, w164, w149, w150, 0.0) -> (w151:cluster{dbl, dbl, dbl, dbl, dbl})  [unwired: 1 in]
            n102 = Divide(x=20, y=w175) -> (x/y=w173:sgl)
            n103 = Bundle("X"=w143, "Y"=w144) -> (w147:cluster{"X":sgl, "Y":sgl})  [unwired: 1 in]
            n104 = call "IMAQ Convert Rectangle to ROI (Polygon)"("Rectangle"=w151) -> ("ROI Descriptor"=w153:T17)  [unwired: 7 in, 2 out]
            n105 = property on="Image Out" class="ImageControl"("Image Center Position"=w147) -> ()  [unwired: 2 in, 2 out]
            n106 = property on="Image Preview" class="ImageControl"("ROI"=w153) -> ()  [unwired: 2 in, 2 out]
            n107 = Bundle("Application Font", w173, w169, w169, w169, w169, w169, TRUE, w171) -> (w168:T18)  [unwired: 1 in]
            n108 = Bundle(w171, w168, w171, w171) -> (w125:T19)  [unwired: 1 in]
            n109 = local read "Image Out"() -> (w124:T8)
            n110 = property on="Image Out" class="ImageControl"() -> ("ZoomInteger"=w123:cluster{"X":i32, "Y":i32})  [unwired: 2 in, 2 out]
            n111 = property on="Image Out" class="ImageControl"() -> ("ROI"=w127:T12)  [unwired: 2 in, 2 out]
            n112 = Unbundle By Name(w127) -> ("Contours"=w128:T13)
            n113 = local read "No Image\n File"() -> (w119:path)
            n114 = local read "Image File"() -> (w118:path)
            n115 = call "IMAQ Clear Overlay"("Image"=w124) -> ("Image Out"=w141:T8)  [unwired: 9 in, 1 out]
            n116 = Initialize Array(0) -> (w130:i32[])  [unwired: 1 in]
            n117 = Array Size(array=w128) -> (size(s)=w129:i32)
            n118 = Unbundle(w123) -> ("X"=w122:i32)  [unwired: 1 out]
            n119 = Equal?(x=w119, y=w118) -> (x = y?=w117:bool)
            n120 = local write "Zoom"(w122) -> ()
            n121 = Build Array(0.505025, 0.252522, 0.127742, 0.050345, 0.031129) -> (w137:dbl[])
            n122 = Array Subset(array=w137, index="Magnification", length=1) -> (w139:dbl[])
            n123 = case shown="True" w117 {
              tunnel: w120 -> [w198 _]
              frame False {
                n124 = local write "Image Center X"(w198) -> ()
              }
              frame True {
              }
            }
            n125 = To Double Precision Float(number=w139) -> (double precision float=w140:dbl[])
            n126 = for {
              N: w129 -> [_]
              shift-right: [w223] -> _
              shift-left: w128 -> [w223]
              shift-right: [w199] -> w114
              shift-left: w130 -> [w221]
              tunnel: w140 -> [w220]
              shift-right: [w217] -> _
              shift-left: w141 -> [w219]
              tunnel: w125 -> [w213]
              i -> [w216]
              n127 = Index Array(array=w223, index=w216) -> (element=w232:T20)
              n128 = Unbundle(w232) -> ("Points"=w231:i32[])  [unwired: 2 out]
              n129 = Array To Cluster(array=w231) -> (cluster=w230:T21)
              n130 = Unbundle(w230) -> ("Points[0]"=w212:i32, "Points[1]"=w209:i32, "Points[2]"=w222:i32, "Points[3]"=w228:i32)  [unwired: 5 out]
              n131 = Add(x=w212, y=10) -> (x+y=w210:i32)
              n132 = Subtract(x=w209, y=w228) -> (x-y=w227:i32)
              n133 = Subtract(x=w212, y=w222) -> (x-y=w229:i32)
              n134 = Square(x=w227) -> (x^2=w225:i32)
              n135 = Square(x=w229) -> (x^2=w226:i32)
              n136 = Add(x=w226, y=w225) -> (x+y=w224:i32)
              n137 = Square Root(x=w224) -> (sqrt(x)=w203:dbl)
              n138 = Multiply(x=w203, y=0.5) -> (x*y=w206:dbl)
              n139 = Add(x=w206, y=w209) -> (x+y=w208:dbl)
              n140 = Bundle(w210, w208) -> (w218:cluster{i32, dbl})  [unwired: 1 in]
              n141 = Multiply(x=w203, y=w220) -> (x*y=w202:dbl[])
              n142 = Index Array(array=w202) -> (element=w215:dbl)  [unwired: 1 in]
              n143 = Number To Fractional String(number=w215, precision (6)=0) -> (F-format string=w214:string)  [unwired: 2 in]
              n144 = call "IMAQ Overlay Text"("BG Color (Transparent)"=u32 0, "Text Color (black)"=u32 16448250, "Font, Size & Style"=w213, "String"=w214, "Origin"=w218, "Image"=w219) -> ("Image Out"=w217:T8)  [unwired: 4 in, 1 out]
              n145 = Build Array (concatenate)(w221, w202) -> (w200:dbl[])
              n146 = To Long Integer(number=w200) -> (32bit integer=w199:i32[])
            }
            "Distances" <- w114
            n147 = Add Array Elements(numeric array=w114) -> (sum=w126:i32)
            n148 = local write "Total Width"(w126) -> ()
          }
        }
        n149 = Unbundle By Name(w106) -> ("Manual-Temp"=w111:bool, "Manual-Width"=w110:bool, "Manuel-Length"=w109:bool, "Manuel-Dielectric"=w108:bool, "Manual Comments"=w107:bool)
        n150 = stacked-sequence {
          tunnel: w111 -> [w573 _ _]
          tunnel: w110 -> [_ w582 _]
          tunnel: w109 -> [_ _ w598]
          tunnel: w108 -> [_ _ w595]
          tunnel: w107 -> [_ _ w594]
          frame #0 {
            n151 = local read "Rec: Temp"() -> (w572:dbl)
            n152 = case shown="False" w573 {
              tunnel: w572 -> [w578 _]
              frame False {
                n153 = local read "Rec: Temp"() -> (w576:dbl)
                n154 = property on="New: Temp" class="DigNum (strict)"("DisabledEnum"=1) -> ()  [unwired: 2 in, 2 out]
                n155 = Equal To 0?(x=w576) -> (x = 0?=w577:bool)
                n156 = local write "New: Temp"(w578) -> ()
                n157 = case shown="True" w577 {
                  tunnel: [w579 w580] -> w574
                  tunnel: w576 -> [w579 _]
                  frame False {
                  }
                  frame True {
                    n158 = local read "Room Temp"() -> (w580:dbl)
                  }
                }
                n159 = local write "Rec: Temp"(w574) -> ()
                n160 = local write "New: Temp"(w574) -> ()
              }
              frame True {
                n161 = property on="New: Temp" class="DigNum (strict)"("DisabledEnum"=0) -> ()  [unwired: 2 in, 2 out]
              }
            }
          }
          frame #1 {
            n162 = case shown="True" w582 {
              frame False {
                n163 = property on="New: Width" class="DigNum (strict)"("DisabledEnum"=1) -> ()  [unwired: 2 in, 2 out]
              }
              frame True {
                n164 = property on="New: Width" class="DigNum (strict)"("DisabledEnum"=0) -> ()  [unwired: 2 in, 2 out]
              }
            }
            n165 = local read "Total Width"() -> (w588:dbl)
            n166 = Equal To 0?(x=w588) -> (x = 0?=w585:bool)
            n167 = local read "Rec: Width"() -> (w586:dbl)
            n168 = Not(x=w582) -> (.not. x?=w584:bool)
            n169 = Or(x=w585, y=w582) -> (x .or. y?=w587:bool)
            n170 = And(x=w585, y=w584) -> (x .and. y?=w583:bool)
            n171 = case shown="True" w583 {
              tunnel: w586 -> [_ w591]
              frame False {
              }
              frame True {
                n172 = local write "New: Width"(w591) -> ()
              }
            }
            n173 = case shown="True" w587 {
              tunnel: w588 -> [w592 _]
              frame False {
                n174 = local write "New: Width"(w592) -> ()
              }
              frame True {
                n175 = property on="New: Width" class="DigNum (strict)"("DisabledEnum"=0) -> ()  [unwired: 2 in, 2 out]
              }
            }
          }
          frame #2 {
            n176 = local read "Rec: Length"() -> (w599:dbl)
            n177 = case shown="False" w598 {
              tunnel: w599 -> [w607 _]
              frame False {
                n178 = local write "New: Length"(w607) -> ()
                n179 = property on="New: Length" class="DigNum (strict)"("DisabledEnum"=1) -> ()  [unwired: 2 in, 2 out]
              }
              frame True {
                n180 = property on="New: Length" class="DigNum (strict)"("DisabledEnum"=0) -> ()  [unwired: 2 in, 2 out]
              }
            }
            n181 = local read "Comments:"() -> (w596:string)
            n182 = local read "Rec: Dielectric (d)"() -> (w597:dbl)
            n183 = case shown="False" w594 {
              tunnel: w596 -> [w601 _]
              frame False {
                n184 = local write "New: Comments"(w601) -> ()
                n185 = property on="New: Comments" class="Str"("DisabledEnum"=1) -> ()  [unwired: 2 in, 2 out]
              }
              frame True {
                n186 = property on="New: Comments" class="Str"("DisabledEnum"=0) -> ()  [unwired: 2 in, 2 out]
              }
            }
            n187 = case shown="False" w595 {
              tunnel: w597 -> [w604 _]
              frame False {
                n188 = local write "New: Dielectric"(w604) -> ()
                n189 = property on="New: Dielectric" class="DigNum (strict)"("DisabledEnum"=1) -> ()  [unwired: 2 in, 2 out]
              }
              frame True {
                n190 = property on="New: Dielectric" class="DigNum (strict)"("DisabledEnum"=0) -> ()  [unwired: 2 in, 2 out]
              }
            }
          }
        }
        n191 = property on="Next File" class="Bool (strict)"("Value"=w93) -> (error out=w102:errorcluster)  [unwired: 2 in, 1 out]
        n192 = property on="Previous File" class="Bool (strict)"(error in=w102, "Value"=w93) -> (error out=w101:errorcluster)  [unwired: 1 in, 1 out]
        n193 = property on="Save" class="Bool (strict)"(error in=w101, "Value"=w93) -> (error out=w100:errorcluster)  [unwired: 1 in, 1 out]
        n194 = property on="Export" class="Bool (strict)"("Value"=w93) -> ()  [unwired: 2 in, 2 out]
        n195 = property on="Save Next" class="Bool (strict)"(error in=w100, "Value"=w93) -> (error out=w99:errorcluster)  [unwired: 1 in, 1 out]
        n196 = property on="Discard" class="Bool (strict)"(error in=w99, "Value"=w93) -> (error out=w98:errorcluster)  [unwired: 1 in, 1 out]
        n197 = property on="Save Lines" class="Bool (strict)"(error in=w98, "Value"=w93) -> ()  [unwired: 1 in, 2 out]
        n198 = property on="Close" class="Bool (strict)"("Value"=w93) -> ()  [unwired: 2 in, 2 out]
        n199 = property on="Disable Flag" class="Bool (strict)"("Value"=w93) -> ()  [unwired: 2 in, 2 out]
        n200 = Cluster To Array(cluster=w92) -> (array=w112:bool[])
        n201 = call "Next State.vi"("Buttons []"=w112, "States []"=w113) -> ("Enum"=w105:T2)
        n202 = event shown="[7] \"Lin-Trans Slider\": Value Change" {
          selector: _ -> [_ _ _ _ _ _ _ _ _ _ _ _ _]
          dyn-events: _ -> [_ _ _ _ _ _ _ _ _ _ _ _ _]
          timeout: 5 -> [_ _ _ _ _ _ _ _ _ _ _ _ _]
          tunnel: w105 -> [w452 _ _ _ _ _ _ _ _ _ _ _ _]
          tunnel: [w452 MegaAwesome_States."Re-Calculated Values" MegaAwesome_States."Re-Calculated Values" MegaAwesome_States."Re-Calculated Values" MegaAwesome_States."Re-Calculated Values" MegaAwesome_States."Calculated Values" MegaAwesome_States."Re-Calculated Values" MegaAwesome_States."Re-Calculated Values" MegaAwesome_States."Calculated Values" MegaAwesome_States."Re-Calculated Values" MegaAwesome_States."Re-Calculated Values" MegaAwesome_States."Read Data" MegaAwesome_States."Read Data"] -> w104
          tunnel: w96 -> [w451 w453 w455 w457 w459 w461 w463 w488 w513 w518 w542 _ w570]
          tunnel: [w451 w453 w455 w457 w459 w461 w463 w488 w513 w518 w542 w561 w570] -> w95
          tunnel: w94 -> [_ _ _ _ _ _ _ _ _ _ _ w560 _]
          tunnel: w92 -> [_ _ _ _ _ _ _ _ _ _ _ _ _]
          event Timeout {
            n203 = event-data() -> ()  [unwired: 1 in, 2 out]
          }
          event "New: Dielectric": Value Change {
            n204 = event-data() -> ()  [unwired: 1 in, 5 out]
          }
          event "New: Length": Value Change {
            n205 = event-data() -> ()  [unwired: 1 in, 5 out]
          }
          event "New: Width": Value Change {
            n206 = event-data() -> ()  [unwired: 1 in, 5 out]
          }
          event "New: Temp": Value Change {
            n207 = event-data() -> ()  [unwired: 1 in, 5 out]
          }
          event "Num Pts Log", "Transport Style Controls", "Num Pts": Value Change {
            n208 = event-data() -> ()  [unwired: 1 in, 5 out]
          }
          event "Sat-Trans Slider": Value Change {
            n209 = event-data() -> ()  [unwired: 1 in, 5 out]
            n210 = local read "Sqrt-Sat"() -> (w487:cluster{dbl[], dbl[]}[])
            n211 = Decimate 1D Array(w487) -> (w471:cluster{dbl[], dbl[]}[], w472:cluster{dbl[], dbl[]}[])
            n212 = local read "Slider Min"() -> (w468:dbl)
            n213 = local read "Sat-Trans Slider"() -> (w466:dbl)
            n214 = Array To Cluster(array=w471) -> (cluster=w486:T22)
            n215 = local read "New: Dielectric"() -> (w481:dbl)
            n216 = local read "Num Pts"() -> (w464:dbl)
            n217 = local read "New: Width"() -> (w483:dbl)
            n218 = local read "New: Length"() -> (w482:dbl)
            n219 = Unbundle(w486) -> ("[0]"=w485:cluster{dbl[], dbl[]})  [unwired: 8 out]
            n220 = Absolute Value(x=w468) -> (abs(x)=w467:dbl)
            n221 = Unbundle(w485) -> (w469:dbl[], w484:dbl[])
            n222 = Add(x=w466, y=w467) -> (x+y=w465:dbl)
            n223 = Array Subset(array=w469, index=w465, length=w464) -> (w479:dbl[])
            n224 = local write "Sat Vg Array-Used"(w479) -> ()
            n225 = Array Subset(array=w484, index=w465, length=w464) -> (w480:dbl[])
            n226 = call "Mobility-Vt-Used Pts_Saturation.vi"("Width"=w483, "Length"=w482, "Dielectric (d)"=w481, "Sat Id Used"=w480, "Vg Used"=w479) -> ("Vt"=w475:dbl, "Mobility"=w476:dbl)  [unwired: 4 in, 1 out]
            n227 = local write "Index-Sat"(w465) -> ()
            n228 = local write "Sat Id-Used"(w480) -> ()
            n229 = Bundle(w479, w480) -> (w473:cluster{dbl[], dbl[]})  [unwired: 1 in]
            n230 = local read "Re-Calculated Values Cluster"() -> (w478:T9)
            n231 = Bundle By Name(cluster=w478, "Mobility-Sat"=w476, "Vt-Sat"=w475) -> (w477:T9)
            n232 = local write "Re-Calculated Values Cluster"(w477) -> ()
            n233 = Build Array (concatenate)(w471, w472, w473) -> (w470:cluster{dbl[], dbl[]}[])
            n234 = local write "Sqrt-Sat"(w470) -> ()
          }
          event "Lin-Trans Slider": Value Change {
            n235 = event-data() -> ()  [unwired: 1 in, 5 out]
            n236 = local read "Sqrt-Lin"() -> (w512:cluster{dbl[], dbl[]}[])
            n237 = Decimate 1D Array(w512) -> (w497:cluster{dbl[], dbl[]}[], w498:cluster{dbl[], dbl[]}[])
            n238 = local read "Slider Min"() -> (w494:dbl)
            n239 = Array To Cluster(array=w497) -> (cluster=w511:T22)
            n240 = local read "Lin-Trans Slider"() -> (w492:dbl)
            n241 = local read "New: Dielectric"() -> (w505:dbl)
            n242 = local read "Num Pts"() -> (w508:dbl)
            n243 = local read "New: Width"() -> (w507:dbl)
            n244 = local read "New: Length"() -> (w506:dbl)
            n245 = local read "Lin Vd"() -> (w489:dbl)
            n246 = Unbundle(w511) -> ("[0]"=w510:cluster{dbl[], dbl[]})  [unwired: 8 out]
            n247 = Absolute Value(x=w494) -> (abs(x)=w493:dbl)
            n248 = Unbundle(w510) -> (w495:dbl[], w509:dbl[])
            n249 = Add(x=w492, y=w493) -> (x+y=w491:dbl)
            n250 = Array Subset(array=w495, index=w491, length=w508) -> (w503:dbl[])
            n251 = local write "Lin-Vg Array-Used"(w503) -> ()
            n252 = Array Subset(array=w509, index=w491, length=w508) -> (w504:dbl[])
            n253 = call "Mobility-Vt-Used Pts_Linear.vi"("Width"=w507, "Length"=w506, "Vd"=w489, "Dielectric (d)"=w505, "Id Used"=w504, "Vg Used"=w503) -> ("Mobility"=w500:dbl)  [unwired: 3 in, 2 out]
            n254 = local write "Index-Lin"(w491) -> ()
            n255 = local write "Lin Id-Used"(w504) -> ()
            n256 = Bundle(w503, w504) -> (w499:cluster{dbl[], dbl[]})  [unwired: 1 in]
            n257 = local read "Re-Calculated Values Cluster"() -> (w502:T9)
            n258 = Bundle By Name(cluster=w502, "Moblitity-Lin"=w500) -> (w501:T9)
            n259 = local write "Re-Calculated Values Cluster"(w501) -> ()
            n260 = Build Array (concatenate)(w497, w498, w499) -> (w496:cluster{dbl[], dbl[]}[])
            n261 = local write "Sqrt-Lin"(w496) -> ()
          }
          event "Image Analysis", "1) Transport": Value Change {
            n262 = event-data() -> ()  [unwired: 1 in, 5 out]
          }
          event "Sat-Log Slider": Value Change {
            n263 = event-data() -> ()  [unwired: 1 in, 5 out]
            n264 = local read "Sat-Log"() -> (w521:cluster{dbl[], dbl[]}[])
            n265 = Decimate 1D Array(w521) -> (w528:cluster{dbl[], dbl[]}[], w529:cluster{dbl[], dbl[]}[])
            n266 = local read "Slider Min"() -> (w525:dbl)
            n267 = Array To Cluster(array=w528) -> (cluster=w538:T22)
            n268 = property on="Sat-Log" class="XYGraph (strict)"("Active Plot"=2, "Plot.Fill/Pt. Color"=u32 6618880, "Plot.Point Style"=11) -> ()  [unwired: 2 in, 2 out]
            n269 = local read "Num Pts Log"() -> (w535:dbl)
            n270 = local read "Sat-Log Slider"() -> (w523:dbl)
            n271 = Unbundle(w538) -> ("[0]"=w537:cluster{dbl[], dbl[]})  [unwired: 8 out]
            n272 = Absolute Value(x=w525) -> (abs(x)=w524:dbl)
            n273 = Unbundle(w537) -> (w526:dbl[], w536:dbl[])
            n274 = Add(x=w523, y=w524) -> (x+y=w520:dbl)
            n275 = Array Subset(array=w526, index=w520, length=w535) -> (w533:dbl[])
            n276 = Array Subset(array=w536, index=w520, length=w535) -> (w534:dbl[])
            n277 = local write "Vg Array-Log-Used"(w533) -> ()
            n278 = local write "IndexLog-Sat"(w520) -> ()
            n279 = Bundle(w533, w534) -> (w519:cluster{dbl[], dbl[]})  [unwired: 1 in]
            n280 = call "STS-Used.vi"("Id Used"=w534, "Vg-Used"=w533) -> ("STS"=w530:dbl)  [unwired: 9 in]
            n281 = local write "Sat Id-Log-Used"(w534) -> ()
            n282 = local read "Re-Calculated Values Cluster"() -> (w532:T9)
            n283 = Bundle By Name(cluster=w532, "STS"=w530) -> (w531:T9)
            n284 = local write "Re-Calculated Values Cluster"(w531) -> ()
            n285 = Build Array (concatenate)(w528, w529, w519) -> (w527:cluster{dbl[], dbl[]}[])
            n286 = local write "Sat-Log"(w527) -> ()
          }
          event "Lin-Log Slider": Value Change {
            n287 = event-data() -> ()  [unwired: 1 in, 5 out]
            n288 = local read "Lin-Log"() -> (w546:cluster{dbl[], dbl[]}[])
            n289 = Decimate 1D Array(w546) -> (w552:cluster{dbl[], dbl[]}[], w553:cluster{dbl[], dbl[]}[])
            n290 = local read "Slider Min"() -> (w549:dbl)
            n291 = Array To Cluster(array=w552) -> (cluster=w559:T22)
            n292 = local read "Num Pts Log"() -> (w556:dbl)
            n293 = property on="Lin-Log" class="XYGraph (strict)"("Active Plot"=2, "Plot.Fill/Pt. Color"=u32 6618880, "Plot.Point Style"=11) -> ()  [unwired: 2 in, 2 out]
            n294 = local read "Lin-Log Slider"() -> (w547:dbl)
            n295 = Unbundle(w559) -> ("[0]"=w558:cluster{dbl[], dbl[]})  [unwired: 8 out]
            n296 = Absolute Value(x=w549) -> (abs(x)=w548:dbl)
            n297 = Unbundle(w558) -> (w550:dbl[], w557:dbl[])
            n298 = Add(x=w547, y=w548) -> (x+y=w545:dbl)
            n299 = Array Subset(array=w550, index=w545, length=w556) -> (w554:dbl[])
            n300 = local write "Lin-Vg Array-Log Used"(w554) -> ()
            n301 = Array Subset(array=w557, index=w545, length=w556) -> (w555:dbl[])
            n302 = local write "IndexLog-Sat"(w545) -> ()
            n303 = Bundle(w554, w555) -> (w544:cluster{dbl[], dbl[]})  [unwired: 1 in]
            n304 = local write "Lin Id-Log Used"(w555) -> ()
            n305 = Build Array (concatenate)(w552, w553, w544) -> (w551:cluster{dbl[], dbl[]}[])
            n306 = local write "Lin-Log"(w551) -> ()
          }
          event "Index Array": Value Change {
            n307 = event-data() -> ()  [unwired: 1 in, 5 out]
            n308 = Strip Path(path=w560) -> (stripped path=w566:path)  [unwired: 1 out]
            n309 = local write "Transfer Folder"(w566) -> ()
            n310 = List Folder(path=w566) -> (filenames=w562:string[])  [unwired: 3 in, 3 out]
            n311 = local read "Index Array"() -> (w561:u16)
            n312 = Path To String(path=w566) -> (string=w567:string)
            n313 = Index Array(array=w562, index=w561) -> (element=w568:string)
            n314 = Concatenate Strings(w567, "\\", w568) -> (w564:string)
            n315 = String To Path(string=w564) -> (path=w563:path)
            n316 = local write "Transfer File"(w563) -> ()
          }
          event "Transfer File": Value Change {
            n317 = event-data() -> ()  [unwired: 1 in, 5 out]
          }
        }
      }
      frame "Read Data" {
        n318 = call "IMAQ Dispose"("All Images? (No)"=TRUE) -> ()  [unwired: 5 in, 1 out]
        n319 = case shown="True" "Disable Flag" {
          tunnel: w617 -> [_ w642]
          tunnel: [w638 w639] -> w616
          tunnel: w614 -> [w638 _]
          frame False {
          }
          frame True {
            n320 = local read "Transfer Folder"() -> (w641:path)
            n321 = List Folder(path=w641) -> (filenames=w643:string[])  [unwired: 3 in, 3 out]
            n322 = Index Array(array=w643, index=w642) -> (element=w640:string)
            n323 = Build Path(base path=w641, name or relative path=w640) -> (appended path=w639:path)
            n324 = local write "Transfer File"(w639) -> ()
          }
        }
        n325 = call "Recorded Values.vi"("Path"=w616) -> ("Recorded Char"=→"Recorded Values Cluster":T9, "Recorded Prop"=w629:T1, "Fabrication Prop"=w627:T4)  [unwired: 8 in]
        n326 = Strip Path(path=w616) -> (stripped path=w626:path, name=w625:string)
        n327 = local write "Fabrication Prop"(w627) -> ()
        n328 = local write "Recorded Prop"(w629) -> ()
        n329 = Unbundle By Name(w629) -> ("Date Recorded"=→"Date Recorded":string, "Index"=w628:string, "Length"=w622:dbl, "Width"=w621:dbl)  [unwired: 1 out]
        n330 = Unbundle By Name(w629) -> ("Sample Temp"=w631:dbl)
        n331 = Unbundle By Name(w627) -> ("Dielectric (nm)"=w623:dbl, "Comments"=w624:string, "Date Created"=→"Date Created":string)
        n332 = List Folder(path=w626) -> (filenames=w620:string[])  [unwired: 3 in, 3 out]
        n333 = local write "Rec: Dielectric (d)"(w623) -> ()
        n334 = local write "Index"(w628) -> ()
        n335 = local write "Rec: Length"(w622) -> ()
        n336 = local write "Rec: Width"(w621) -> ()
        n337 = Equal To 0?(x=w631) -> (x = 0?=w634:bool)
        n338 = Number To Decimal String(number=w631) -> (decimal integer string=w635:string)  [unwired: 1 in]
        n339 = local write "Comments:"(w624) -> ()
        n340 = Search 1D Array(1D array=w620, element=w625) -> (index of element=w619:i32)  [unwired: 1 in]
        n341 = Equal?(x="", y=w635) -> (x = y?=w633:bool)
        n342 = Index Array(array=w620, index=w619) -> (element=→"Data Name:":string)
        n343 = local write "New: Width"(w621) -> ()
        n344 = local write "New: Length"(w622) -> ()
        n345 = local write "Index Array"(w619) -> ()
        n346 = Or(x=w634, y=w633) -> (x .or. y?=w632:bool)
        n347 = local write "New: Dielectric"(w623) -> ()
        n348 = case shown="True" w632 {
          tunnel: [w644 w645] -> w613
          tunnel: w631 -> [w644 _]
          frame False {
          }
          frame True {
            n349 = local read "Room Temp"() -> (w645:dbl)
          }
        }
        n350 = local write "New: Temp"(w613) -> ()
        n351 = Bundle By Name(cluster=w629, "Sample Temp"=w613) -> (w630:T1)
        n352 = local write "Rec: Temp"(w613) -> ()
        n353 = local write "Recorded Prop"(w630) -> ()
      }
      frame "Calculated Values" {
        n354 = case shown="False" w653 {
          selector: w653 -> [w726 _]
          tunnel: w662 -> [w725 w735]
          tunnel: w651 -> [w724 w733]
          tunnel: w650 -> [w727 w732]
          tunnel: [w723 w729] -> w647
          tunnel: [w722 w728] -> w646
          frame False {
            n355 = call "TRF to TSP Plot_09_21_12a_JW.vi"("Plot Transport"=w726, "No Transport File"=w727, "Transport Folder"=w724, "Transfer File"=w725) -> ("Transport"=w722:cluster{ext[], ext[]}[], "Transport File"=w723:path)  [unwired: 5 in, 1 out]
          }
          frame True {
            n356 = call "TRF to TSP Plot_09_21_12a_JW.vi"("Transport Graph Properties"="Transport Style Controls", "No Transport File"=w732, "Transport Folder"=w733, "Transfer File"=w735) -> ("Transport"=w728:cluster{ext[], ext[]}[], "Transport File"=w729:path, "Transport Name"=→"Transport Name:":string)  [unwired: 5 in]
            n357 = Array Size(array=w728) -> (size(s)=w734:i32)
            n358 = for {
              N: w734 -> [_]
              tunnel: "Transport Style Controls" -> [w739]
              i -> [w738]
              n359 = Unbundle By Name(w739) -> ("Transport Line Size"=w736:u16, "Transport Line Color"=w737:u32)
              n360 = property on="Transport" class="XYGraph (strict)"("Active Plot"=w738, "Plot.Plot Color"=w737, "Plot.Line Width"=w736) -> ()  [unwired: 2 in, 2 out]
            }
          }
        }
        "Transport\nFile" <- w647
        "Transport" <- w646
        n361 = case shown="True" w652 {
          tunnel: w681 -> [_ w711]
          tunnel: w680 -> [w702 w716]
          tunnel: w662 -> [_ w715]
          frame False {
            n362 = call "Vision Acquisition2"("Image Path"=w702) -> ("Image Out"=w701:T8)  [unwired: 25 in, 1 out]
            n363 = local write "Image Out"(w701) -> ()
            n364 = local write "Image Preview"(w701) -> ()
          }
          frame True {
            n365 = local read "Image Center X"() -> (w704:i32)
            n366 = call "Image from TRF Display.vi"("Image Center X"=w704, "No Image File"=w716, "Image Folder"=w711, "Transfer File"=w715) -> ("Image Preview"=w712:T8, "Image Out"=w713:T8, "Image File"=w714:path, "Image Name"=→"Image Name":string, "ROI File"=w708:path)  [unwired: 3 in]
            n367 = invoke on="Image Out" class="ImageControl" method="Clear ROI"() -> ()  [unwired: 3 in, 3 out]
            n368 = local write "Image File"(w714) -> ()
            n369 = local write "Image Out"(w713) -> ()
            n370 = local write "Image Preview"(w712) -> ()
            n371 = call <vilib>:"Check if File or Folder Exists.vi"("path"=w708) -> ("file or folder exists?"=w709:bool, "dup path"=w710:path)  [unwired: 8 in, 1 out]
            n372 = case shown="True" w709 {
              tunnel: w710 -> [_ w717]
              frame False {
              }
              frame True {
                n373 = Read from Text File(file (use dialog)=w717) -> (text=w721:string)  [unwired: 3 in, 3 out]
                n374 = property on="Image Out" class="ImageControl"() -> ("ROI"=w718:T12)  [unwired: 2 in, 2 out]
                n375 = Unflatten From String(type=w718, binary string=w721) -> (value=w719:T12, error out=w720:errorcluster)  [unwired: 3 in, 1 out]
                n376 = property on="Image Out" class="ImageControl"(error in=w720, "ROI"=w719) -> ()  [unwired: 1 in, 2 out]
              }
            }
            n377 = local read "Image Center X"() -> (w705:i32)
            n378 = Bundle("Image Center X"=w705, 0) -> (w707:cluster{"Image Center X":i32, i32})  [unwired: 1 in]
            n379 = property on="Image Out" class="ImageControl"("Image Center Position"=w707) -> ()  [unwired: 2 in, 2 out]
          }
        }
        n380 = local read "Recorded Prop"() -> (w683:T1)
        n381 = local read "Fabrication Prop"() -> (w690:T4)
        n382 = local read "Calculated Values Cluster"() -> (w700:T9)
        n383 = call "Mobility-Vt Calculator-File.vi"("NumPts"=w685, "Path"=w662) -> ("Used Points"=w678:T23, "Graph Cluster"=w668:T24, "Lin Vd"=w648:dbl, "Output"=w698:T25)  [unwired: 6 in]
        n384 = call "STS Calculator-File.vi"("NumPts"=w684, "Path"=w662) -> ("Used Points"=w673:T26, "XY Graph-Sat"=w656:cluster{dbl[], dbl[]}[], "XY Graph-Lin"=w649:cluster{dbl[], dbl[]}[], "Ouput"=w693:cluster{"STS-Sat":dbl, "STS-Lin":dbl})  [unwired: 6 in]
        n385 = Unbundle By Name(w690) -> ("Dielectric (nm)"=w688:dbl)
        n386 = Unbundle By Name(w683) -> ("Sample Temp"=w682:dbl)
        n387 = Unbundle By Name(w698) -> ("Mobility-Sat"=w697:dbl, "Vt-Sat"=w689:dbl, "Mobility-Lin"=w696:dbl, "Off I-Sat"=w695:dbl, "On/Off I-Sat"=w694:dbl)  [unwired: 1 out]
        n388 = local write "Lin Vd"(w648) -> ()
        n389 = Unbundle By Name(w693) -> ("STS-Sat"=w687:dbl)  [unwired: 1 out]
        n390 = local write "Sat-Log"(w656) -> ()
        n391 = local write "Lin-Log"(w649) -> ()
        n392 = call "Trap Density_VT.vi"("VT"=w689, "Dielectric"=w688) -> ("Trap Density-VT"=w692:dbl)
        n393 = call "Trap Density_STS.vi"("Temp (T) [K]"=w682, "S.T.S. (S)"=w687, "Dielectric"=w688) -> ("Trap Density (N)"=w691:dbl)  [unwired: 8 in]
        n394 = Bundle By Name(cluster=w700, "Mobility-Sat"=w697, "Moblitity-Lin"=w696, "On/Off"=w694, "Off Current"=w695, "Vt-Sat"=w689, "STS"=w687, "Trap Density-VT"=w692, "Trap Density-STS"=w691) -> (w699:T9)
        n395 = Unbundle By Name(w673) -> ("Sat Vg Used"=w672:dbl[], "Sat Log(Id) Used"=w671:dbl[], "Lin Vg Used"=w670:dbl[], "Lin Log(Id) Used"=w669:dbl[], "STS Index-Sat"=w654:dbl, "STS Index-Lin"=w655:dbl)
        n396 = Unbundle By Name(w678) -> ("Sat Vg Used"=w677:dbl[], "Sat Sqrt(Id) Used"=w676:dbl[], "Lin Vg Used"=w675:dbl[], "Lin Sqrt(Id) Used"=w674:dbl[], "Index-Lin"=w664:dbl, "Index-Sat"=w663:dbl)
        n397 = local write "Vg Array-Log-Used"(w672) -> ()
        n398 = local write "Sat Id-Log-Used"(w671) -> ()
        n399 = local write "Lin-Vg Array-Log Used"(w670) -> ()
        n400 = local write "Lin Id-Log Used"(w669) -> ()
        n401 = local write "IndexLog-Sat"(w654) -> ()
        n402 = local write "Index-Lin"(w655) -> ()
        n403 = local write "Calculated Values Cluster"(w699) -> ()
        n404 = local write "Sat Vg Array-Used"(w677) -> ()
        n405 = local write "Sat Id-Used"(w676) -> ()
        n406 = local write "Lin-Vg Array-Used"(w675) -> ()
        n407 = local write "Lin Id-Used"(w674) -> ()
        n408 = local write "Index-Sat"(w663) -> ()
        n409 = local write "Index-Lin"(w664) -> ()
        n410 = local write "Lin-Log Slider"(w655) -> ()
        n411 = local write "Sat-Log Slider"(w654) -> ()
        n412 = local write "Sat-Trans Slider"(w663) -> ()
        n413 = local write "Lin-Trans Slider"(w664) -> ()
        n414 = Unbundle By Name(w668) -> ("Raw Sat"=w661:cluster{dbl[], dbl[]}[], "Sqrt Sat"=w665:cluster{dbl[], dbl[]}[], "Raw Lin"=w667:cluster{dbl[], dbl[]}[], "Sqrt Lin"=w666:cluster{dbl[], dbl[]}[])
        n415 = Index Array(array=w661) -> (element=w660:cluster{dbl[], dbl[]})  [unwired: 1 in]
        n416 = Unbundle(w660) -> (w659:dbl[])  [unwired: 1 out]
        n417 = Array Max & Min(array=w659) -> (max value=w658:dbl, min value=w657:dbl)  [unwired: 2 out]
        n418 = property on="Sat-Trans Slider" class="Slide (strict)"("Scale.Maximum"=w658, "Scale.Minimum"=w657) -> ()  [unwired: 2 in, 2 out]
        n419 = property on="Lin-Trans Slider" class="Slide (strict)"("Scale.Maximum"=w658, "Scale.Minimum"=w657) -> ()  [unwired: 2 in, 2 out]
        n420 = property on="Sat-Log Slider" class="Slide (strict)"("Scale.Maximum"=w658, "Scale.Minimum"=w657) -> ()  [unwired: 2 in, 2 out]
        n421 = property on="Lin-Log Slider" class="Slide (strict)"("Scale.Maximum"=w658, "Scale.Minimum"=w657) -> ()  [unwired: 2 in, 2 out]
        n422 = local write "Slider Max"(w658) -> ()
        n423 = local write "Slider Min"(w657) -> ()
        n424 = local write "Raw- Sat"(w661) -> ()
        n425 = local write "Raw- Lin"(w667) -> ()
        n426 = local write "Sqrt-Sat"(w665) -> ()
        n427 = local write "Sqrt-Lin"(w666) -> ()
      }
      frame "Re-Calculated Values" {
        n428 = local read "Vg Array-Log-Used"() -> (w748:dbl[])
        n429 = local read "Sat Vg Array-Used"() -> (w756:dbl[])
        n430 = local read "Lin-Vg Array-Used"() -> (w762:dbl[])
        n431 = local read "Sat Id-Log-Used"() -> (w747:dbl[])
        n432 = local read "New: Dielectric"() -> (w760:dbl)
        n433 = local read "New: Dielectric"() -> (w745:dbl)
        n434 = local read "New: Length"() -> (w759:dbl)
        n435 = local read "New: Length"() -> (w755:dbl)
        n436 = local read "New: Width"() -> (w758:dbl)
        n437 = local read "New: Width"() -> (w754:dbl)
        n438 = local read "Lin Id-Used"() -> (w761:dbl[])
        n439 = local read "Sat Id-Used"() -> (w753:dbl[])
        n440 = local read "Re-Calculated Values Cluster"() -> (w764:T9)
        n441 = local read "New: Dielectric"() -> (w744:dbl)
        n442 = local read "New: Temp"() -> (w743:dbl)
        n443 = local read "Lin Vd"() -> (w740:dbl)
        n444 = call "Mobility-Vt-Used Pts_Saturation.vi"("Width"=w754, "Length"=w755, "Dielectric (d)"=w745, "Sat Id Used"=w753, "Vg Used"=w756) -> ("Vt"=w751:dbl, "Mobility"=w752:dbl)  [unwired: 4 in, 1 out]
        n445 = call "STS-Used.vi"("Id Used"=w747, "Vg-Used"=w748) -> ("STS"=w746:dbl)  [unwired: 9 in]
        n446 = call "Mobility-Vt-Used Pts_Linear.vi"("Width"=w758, "Length"=w759, "Vd"=w740, "Dielectric (d)"=w760, "Id Used"=w761, "Vg Used"=w762) -> ("Mobility"=w757:dbl)  [unwired: 3 in, 2 out]
        n447 = call "Trap Density_VT.vi"("VT"=w751, "Dielectric"=w745) -> ("Trap Density-VT"=w750:dbl)
        n448 = call "Trap Density_STS.vi"("Temp (T) [K]"=w743, "S.T.S. (S)"=w746, "Dielectric"=w744) -> ("Trap Density (N)"=w742:dbl)  [unwired: 8 in]
        n449 = Bundle By Name(cluster=w764, "Mobility-Sat"=w752, "Moblitity-Lin"=w757, "Vt-Sat"=w751, "STS"=w746, "Trap Density-VT"=w750, "Trap Density-STS"=w742) -> (w763:T9)
        n450 = local write "Re-Calculated Values Cluster"(w763) -> ()
      }
      frame "Next File" {
        n451 = call "IMAQ Dispose"("All Images? (No)"=TRUE) -> ()  [unwired: 5 in, 1 out]
        n452 = Strip Path(path=w781) -> (stripped path=w772:path, name=w779:string)
        n453 = local write "Transfer Folder"(w772) -> ()
        n454 = List Folder(path=w772) -> (filenames=w766:string[])  [unwired: 3 in, 3 out]
        n455 = Array Size(array=w766) -> (size(s)=w778:i32)
        n456 = Search 1D Array(1D array=w766, element=w779) -> (index of element=w776:i32)  [unwired: 1 in]
        n457 = Decrement(x=w778) -> (x-1=w777:i32)
        n458 = Equal?(x=w777, y=w776) -> (x = y?=w775:bool)
        n459 = case shown="True" w775 {
          tunnel: w768 -> [w783 _]
          tunnel: [w782 0] -> w767
          frame False {
            n460 = Increment(x=w783) -> (x+1=w782:i32)
          }
          frame True {
          }
        }
        n461 = Path To String(path=w772) -> (string=w773:string)
        n462 = Index Array(array=w766, index=w767) -> (element=w774:string)
        n463 = Concatenate Strings(w773, "\\", w774) -> (w770:string)
        n464 = String To Path(string=w770) -> (path=w769:path)
        n465 = local write "Transfer File"(w769) -> ()
      }
      frame "Previous File" {
        n466 = call "IMAQ Dispose"("All Images? (No)"=TRUE) -> ()  [unwired: 5 in, 1 out]
        n467 = Strip Path(path=w792) -> (stripped path=w789:path, name=w800:string)
        n468 = local write "Transfer Folder"(w789) -> ()
        n469 = List Folder(path=w789) -> (filenames=w793:string[])  [unwired: 3 in, 3 out]
        n470 = Array Size(array=w793) -> (size(s)=w787:i32)
        n471 = Search 1D Array(1D array=w793, element=w800) -> (index of element=w799:i32)  [unwired: 1 in]
        n472 = Decrement(x=w787) -> (x-1=w786:i32)
        n473 = Equal To 0?(x=w799) -> (x = 0?=w798:bool)
        n474 = case shown="True" w798 {
          tunnel: w791 -> [w803 _]
          tunnel: [w802 w804] -> w790
          tunnel: w786 -> [_ w804]
          frame False {
            n475 = Decrement(x=w803) -> (x-1=w802:i32)
          }
          frame True {
          }
        }
        n476 = Path To String(path=w789) -> (string=w788:string)
        n477 = Index Array(array=w793, index=w790) -> (element=w797:string)
        n478 = Concatenate Strings(w788, "\\", w797) -> (w795:string)
        n479 = String To Path(string=w795) -> (path=w794:path)
        n480 = local write "Transfer File"(w794) -> ()
      }
      frame "Discard File" {
        n481 = flat-sequence {
          tunnel: w810 -> [w813]
          tunnel: [w813] -> w809
          tunnel: [w812] -> w806
          tunnel: w809 -> [w825]
          tunnel: w806 -> [w818]
          tunnel: [w817] -> w805
          frame #0 {
            n482 = Strip Path(path=w813) -> (stripped path=w816:path, name=w815:string)
            n483 = List Folder(path=w816) -> (filenames=w814:string[])  [unwired: 3 in, 3 out]
            n484 = Search 1D Array(1D array=w814, element=w815) -> (index of element=w812:i32)  [unwired: 1 in]
          }
          frame #1 {
            n485 = Strip Path(path=w825) -> (stripped path=w826:path, name=w824:string)
            n486 = String Subset(string=w824, offset (0)=0, length (rest)=1) -> (substring=w821:string)
            n487 = Equal?(x=w821, y="X") -> (x = y?=w819:bool)
            n488 = case shown="True" w819 {
              tunnel: w826 -> [w833 _]
              tunnel: w825 -> [w829 _]
              tunnel: w824 -> [w828 _]
              tunnel: w818 -> [w827 w837]
              tunnel: [w827 w836] -> w817
              frame False {
                n489 = Path To String(path=w833) -> (string=w832:string)
                n490 = Concatenate Strings(w832, "\\", "X_", w828) -> (w831:string)
                n491 = String To Path(string=w831) -> (path=w830:path)
                n492 = Move(source path=w829, 10:w830) -> ()  [unwired: 3 in, 3 out]
              }
              frame True {
                n493 = Increment(x=w837) -> (x+1=w836:i32)
              }
            }
          }
        }
        n494 = property on="Disable Flag" class="Bool (strict)"("Value"=TRUE) -> ()  [unwired: 2 in, 2 out]
        n495 = call "IMAQ Dispose"("All Images? (No)"=TRUE) -> ()  [unwired: 5 in, 1 out]
      }
      frame "Save" {
        n496 = stacked-sequence {
          seq-local: [w853 _] -> [_ w1350]
          seq-local: [w852 _] -> [_ w1348]
          tunnel: w845 -> [w854 w1351]
          frame #0 {
            # "Saves each Re-calculated parameter in sequence"
            n497 = stacked-sequence {
              tunnel: [_ _ _ _ _ _ _ _ _ _ _ _ _ w1318] -> w852
              tunnel: w854 -> [w874 _ _ _ _ _ _ _ _ _ _ _ _ _]
              frame #0 {
                n498 = call-poly <vilib>:"Read From Spreadsheet File.vi"("file path (dialog if empty)"=w874) -> ("all rows"=w873:string[][])  [unwired: 6 in, 4 out]
                n499 = Array Size(array=w873) -> (size(s)=w878:i32[])
                n500 = Array Subset(array=w873, index (row)=0, index (col)=0, length (col)=3) -> (w882:string[][])  [unwired: 1 in]
                n501 = Index Array(array=w878, index=0) -> (element=w876:i32)
                n502 = Reshape Array(w882, w876) -> (w875:string[])
                n503 = Search 1D Array(1D array=w875, element="Dielectric (nm):") -> (index of element=w885:i32)  [unwired: 1 in]
                n504 = Equal?(x=w885, y=-1) -> (x = y?=w884:bool)
                n505 = case shown="False" w884 {
                  tunnel: w873 -> [w893 w897]
                  tunnel: w885 -> [w889 _]
                  tunnel: [w888 w897] -> w883
                  frame False {
                    n506 = local read "Rec: Dielectric (d)"() -> (w895:dbl)
                    n507 = Number To Fractional String(number=w895) -> (F-format string=w890:string)  [unwired: 3 in]
                    n508 = Divide(x=w889, y=3) -> (x/y=w892:dbl)
                    n509 = To Word Integer(number=w892) -> (16bit integer=w891:i16)
                    n510 = Replace Array Subset(array=w893, new element=w890, index (row)=w891, index (col)=1) -> (w888:string[][])
                  }
                  frame True {
                  }
                }
                n511 = local write "Save Array"(w883) -> ()
              }
              frame #1 {
                n512 = local read "Save Array"() -> (w899:string[][])
                n513 = Array Size(array=w899) -> (size(s)=w902:i32[])
                n514 = Array Subset(array=w899, index (row)=0, index (col)=0, length (col)=3) -> (w906:string[][])  [unwired: 1 in]
                n515 = Index Array(array=w902, index=0) -> (element=w900:i32)
                n516 = Reshape Array(w906, w900) -> (w898:string[])
                n517 = Search 1D Array(1D array=w898, element="Comments:") -> (index of element=w909:i32)  [unwired: 1 in]
                n518 = Equal?(x=w909, y=-1) -> (x = y?=w908:bool)
                n519 = case shown="False" w908 {
                  tunnel: w899 -> [w917 w920]
                  tunnel: w909 -> [w914 _]
                  tunnel: [w913 w920] -> w907
                  frame False {
                    n520 = local read "New: Comments"() -> (w912:string)
                    n521 = Divide(x=w914, y=3) -> (x/y=w916:dbl)
                    n522 = To Word Integer(number=w916) -> (16bit integer=w915:i16)
                    n523 = Replace Array Subset(array=w917, new element=w912, index (row)=w915, index (col)=1) -> (w913:string[][])
                  }
                  frame True {
                  }
                }
                n524 = local write "Save Array"(w907) -> ()
              }
              frame #2 {
                n525 = local read "Save Array"() -> (w922:string[][])
                n526 = Array Size(array=w922) -> (size(s)=w925:i32[])
                n527 = Array Subset(array=w922, index (row)=0, index (col)=0, length (col)=3) -> (w929:string[][])  [unwired: 1 in]
                n528 = Index Array(array=w925, index=0) -> (element=w923:i32)
                n529 = Reshape Array(w929, w923) -> (w921:string[])
                n530 = Search 1D Array(1D array=w921, element="Length (um):") -> (index of element=w932:i32)  [unwired: 1 in]
                n531 = Equal?(x=w932, y=-1) -> (x = y?=w931:bool)
                n532 = case shown="False" w931 {
                  tunnel: w922 -> [w942 w945]
                  tunnel: w932 -> [w939 _]
                  tunnel: [w938 w945] -> w930
                  frame False {
                    n533 = local read "New: Length"() -> (w935:dbl)
                    n534 = Divide(x=w939, y=3) -> (x/y=w941:dbl)
                    n535 = Format Value(format string="%#g", value (0)=w935) -> (output string=w936:string)  [unwired: 1 in]
                    n536 = To Word Integer(number=w941) -> (16bit integer=w940:i16)
                    n537 = Replace Array Subset(array=w942, new element=w936, index (row)=w940, index (col)=1) -> (w938:string[][])
                  }
                  frame True {
                  }
                }
                n538 = local write "Save Array"(w930) -> ()
              }
              frame #3 {
                n539 = local read "Save Array"() -> (w947:string[][])
                n540 = Array Size(array=w947) -> (size(s)=w952:i32[])
                n541 = Array Subset(array=w947, index (row)=0, index (col)=0, length (col)=3) -> (w948:string[][])  [unwired: 1 in]
                n542 = Index Array(array=w952, index=0) -> (element=w954:i32)
                n543 = Reshape Array(w948, w954) -> (w946:string[])
                n544 = Search 1D Array(1D array=w946, element="Width (um):") -> (index of element=w957:i32)  [unwired: 1 in]
                n545 = Equal?(x=w957, y=-1) -> (x = y?=w956:bool)
                n546 = case shown="False" w956 {
                  tunnel: w957 -> [w965 _]
                  tunnel: w947 -> [w964 w970]
                  tunnel: [w963 w970] -> w955
                  frame False {
                    n547 = local read "New: Width"() -> (w960:dbl)
                    n548 = Divide(x=w965, y=3) -> (x/y=w967:dbl)
                    n549 = To Word Integer(number=w967) -> (16bit integer=w966:i16)
                    n550 = Format Value(format string="%#g", value (0)=w960) -> (output string=w961:string)  [unwired: 1 in]
                    n551 = Replace Array Subset(array=w964, new element=w961, index (row)=w966, index (col)=1) -> (w963:string[][])
                  }
                  frame True {
                  }
                }
                n552 = local write "Save Array"(w955) -> ()
              }
              frame #4 {
                w980 = "Sample Temp (K):"
                n553 = local read "Save Array"() -> (w972:string[][])
                n554 = Array Size(array=w972) -> (size(s)=w977:i32[])
                n555 = Array Subset(array=w972, index (row)=0, index (col)=0, length (col)=3) -> (w973:string[][])  [unwired: 1 in]
                n556 = Index Array(array=w977, index=0) -> (element=w979:i32)
                n557 = Reshape Array(w973, w979) -> (w971:string[])
                n558 = Search 1D Array(1D array=w971, element=w980) -> (index of element=w983:i32)  [unwired: 1 in]
                n559 = Equal?(x=w983, y=-1) -> (x = y?=w982:bool)
                n560 = case shown="True" w982 {
                  tunnel: w972 -> [w992 w1006]
                  tunnel: w983 -> [w989 _]
                  tunnel: [w988 w1005] -> w981
                  tunnel: w971 -> [_ w1008]
                  tunnel: w980 -> [_ w995]
                  frame False {
                    n561 = local read "New: Temp"() -> (w986:dbl)
                    n562 = Divide(x=w989, y=3) -> (x/y=w991:dbl)
                    n563 = Format Value(format string="%#g", value (0)=w986) -> (output string=w985:string)  [unwired: 1 in]
                    n564 = To Word Integer(number=w991) -> (16bit integer=w990:i16)
                    n565 = Replace Array Subset(array=w992, new element=w985, index (row)=w990, index (col)=1) -> (w988:string[][])
                  }
                  frame True {
                    n566 = local read "New: Temp"() -> (w997:dbl)
                    n567 = Search 1D Array(1D array=w1008, element="Width (um):") -> (index of element=w1002:i32)  [unwired: 1 in]
                    n568 = Divide(x=w1002, y=3) -> (x/y=w1003:dbl)
                    n569 = To Word Integer(number=w1003) -> (16bit integer=w1001:i16)
                    n570 = Format Value(format string="%#g", value (0)=w997) -> (output string=w996:string)  [unwired: 1 in]
                    n571 = Build Array(w995, w996) -> (w999:string[])
                    n572 = Increment(x=w1001) -> (x+1=w1000:i16)
                    n573 = Insert Into Array(array=w1006, index (row)=w1000, new element=w999) -> (w1005:string[][])  [unwired: 1 in]
                  }
                }
                n574 = local write "Save Array"(w981) -> ()
              }
              frame #5 {
                w1018 = "Mobility-Sat (cm^2/Vs):"
                n575 = local read "Save Array"() -> (w1010:string[][])
                n576 = Array Size(array=w1010) -> (size(s)=w1015:i32[])
                n577 = Array Subset(array=w1010, index (row)=0, index (col)=0, length (col)=3) -> (w1011:string[][])  [unwired: 1 in]
                n578 = Index Array(array=w1015, index=0) -> (element=w1017:i32)
                n579 = Reshape Array(w1011, w1017) -> (w1009:string[])
                n580 = Search 1D Array(1D array=w1009, element=w1018) -> (index of element=w1021:i32)  [unwired: 1 in]
                n581 = Equal?(x=w1021, y=-1) -> (x = y?=w1020:bool)
                n582 = case shown="True" w1020 {
                  tunnel: w1010 -> [w1031 w1041]
                  tunnel: w1021 -> [w1028 _]
                  tunnel: [w1027 w1040] -> w1019
                  tunnel: w1009 -> [_ w1038]
                  tunnel: w1018 -> [_ w1036]
                  frame False {
                    n583 = local read "Re-Calculated Values Cluster"() -> (w1024:T9)
                    n584 = Unbundle By Name(w1024) -> ("Mobility-Sat"=w1023:dbl)
                    n585 = Divide(x=w1028, y=3) -> (x/y=w1030:dbl)
                    n586 = To Word Integer(number=w1030) -> (16bit integer=w1029:i16)
                    n587 = Format Value(format string="%#g", value (0)=w1023) -> (output string=w1025:string)  [unwired: 1 in]
                    n588 = Replace Array Subset(array=w1031, new element=w1025, index (row)=w1029, index (col)=1) -> (w1027:string[][])
                  }
                  frame True {
                    n589 = local read "Re-Calculated Values Cluster"() -> (w1035:T9)
                    n590 = Unbundle By Name(w1035) -> ("Mobility-Sat"=w1034:dbl)
                    n591 = Search 1D Array(1D array=w1038, element="Mobility (cm^2/Vs):") -> (index of element=w1044:i32)  [unwired: 1 in]
                    n592 = Divide(x=w1044, y=3) -> (x/y=w1045:dbl)
                    n593 = To Word Integer(number=w1045) -> (16bit integer=w1037:i16)
                    n594 = Format Value(format string="%#g", value (0)=w1034) -> (output string=w1039:string)  [unwired: 1 in]
                    n595 = Build Array(w1036, w1039) -> (w1043:string[])
                    n596 = Replace Array Subset(array=w1041, new element=w1043, index (row)=w1037) -> (w1040:string[][])  [unwired: 1 in]
                  }
                }
                n597 = local write "Save Array"(w1019) -> ()
              }
              frame #6 {
                w1057 = "Mobility-Lin (cm^2/Vs):"
                n598 = local read "Save Array"() -> (w1048:string[][])
                n599 = Array Size(array=w1048) -> (size(s)=w1054:i32[])
                n600 = Array Subset(array=w1048, index (row)=0, index (col)=0, length (col)=3) -> (w1050:string[][])  [unwired: 1 in]
                n601 = Index Array(array=w1054, index=0) -> (element=w1056:i32)
                n602 = Reshape Array(w1050, w1056) -> (w1049:string[])
                n603 = Search 1D Array(1D array=w1049, element=w1057) -> (index of element=w1060:i32)  [unwired: 1 in]
                n604 = Equal?(x=w1060, y=-1) -> (x = y?=w1059:bool)
                n605 = case shown="True" w1059 {
                  tunnel: w1048 -> [w1070 w1078]
                  tunnel: w1060 -> [w1067 _]
                  tunnel: [w1066 w1077] -> w1058
                  tunnel: w1049 -> [_ w1076]
                  tunnel: w1057 -> [_ w1075]
                  frame False {
                    n606 = local read "Re-Calculated Values Cluster"() -> (w1063:T9)
                    n607 = Unbundle By Name(w1063) -> ("Moblitity-Lin"=w1062:dbl)
                    n608 = Divide(x=w1067, y=3) -> (x/y=w1069:dbl)
                    n609 = To Word Integer(number=w1069) -> (16bit integer=w1068:i16)
                    n610 = Format Value(format string="%#g", value (0)=w1062) -> (output string=w1064:string)  [unwired: 1 in]
                    n611 = Replace Array Subset(array=w1070, new element=w1064, index (row)=w1068, index (col)=1) -> (w1066:string[][])
                  }
                  frame True {
                    n612 = local read "Re-Calculated Values Cluster"() -> (w1074:T9)
                    n613 = Unbundle By Name(w1074) -> ("Moblitity-Lin"=w1073:dbl)
                    n614 = Search 1D Array(1D array=w1076, element="Mobility-Sat (cm^2/Vs):") -> (index of element=w1083:i32)  [unwired: 1 in]
                    n615 = Divide(x=w1083, y=3) -> (x/y=w1084:dbl)
                    n616 = To Word Integer(number=w1084) -> (16bit integer=w1082:i16)
                    n617 = Format Value(format string="%#g", value (0)=w1073) -> (output string=w1087:string)  [unwired: 1 in]
                    n618 = Build Array(w1075, w1087) -> (w1080:string[])
                    n619 = Increment(x=w1082) -> (x+1=w1081:i16)
                    n620 = Insert Into Array(array=w1078, index (row)=w1081, new element=w1080) -> (w1077:string[][])  [unwired: 1 in]
                  }
                }
                n621 = local write "Save Array"(w1058) -> ()
              }
              frame #7 {
                w1097 = "On/Off I-Sat:"
                n622 = local read "Save Array"() -> (w1088:string[][])
                n623 = Array Size(array=w1088) -> (size(s)=w1094:i32[])
                n624 = Array Subset(array=w1088, index (row)=0, index (col)=0, length (col)=3) -> (w1090:string[][])  [unwired: 1 in]
                n625 = Index Array(array=w1094, index=0) -> (element=w1096:i32)
                n626 = Reshape Array(w1090, w1096) -> (w1089:string[])
                n627 = Search 1D Array(1D array=w1089, element=w1097) -> (index of element=w1100:i32)  [unwired: 1 in]
                n628 = Equal?(x=w1100, y=-1) -> (x = y?=w1099:bool)
                n629 = case shown="True" w1099 {
                  tunnel: w1088 -> [w1110 w1119]
                  tunnel: w1100 -> [w1107 _]
                  tunnel: [w1106 w1120] -> w1098
                  tunnel: w1089 -> [_ w1117]
                  tunnel: w1097 -> [_ w1115]
                  frame False {
                    n630 = local read "Calculated Values Cluster"() -> (w1103:T9)
                    n631 = Divide(x=w1107, y=3) -> (x/y=w1109:dbl)
                    n632 = Unbundle By Name(w1103) -> ("On/Off"=w1102:dbl)
                    n633 = To Word Integer(number=w1109) -> (16bit integer=w1108:i16)
                    n634 = Format Value(format string="%#g", value (0)=w1102) -> (output string=w1104:string)  [unwired: 1 in]
                    n635 = Replace Array Subset(array=w1110, new element=w1104, index (row)=w1108, index (col)=1) -> (w1106:string[][])
                  }
                  frame True {
                    n636 = local read "Calculated Values Cluster"() -> (w1114:T9)
                    n637 = Unbundle By Name(w1114) -> ("On/Off"=w1113:dbl)
                    n638 = Search 1D Array(1D array=w1117, element="On/Off Current:") -> (index of element=w1123:i32)  [unwired: 1 in]
                    n639 = Divide(x=w1123, y=3) -> (x/y=w1124:dbl)
                    n640 = To Word Integer(number=w1124) -> (16bit integer=w1116:i16)
                    n641 = Format Value(format string="%#g", value (0)=w1113) -> (output string=w1118:string)  [unwired: 1 in]
                    n642 = Build Array(w1115, w1118) -> (w1122:string[])
                    n643 = Replace Array Subset(array=w1119, new element=w1122, index (row)=w1116) -> (w1120:string[][])  [unwired: 1 in]
                  }
                }
                n644 = local write "Save Array"(w1098) -> ()
              }
              frame #8 {
                w1136 = "Off I-Sat (A):"
                n645 = local read "Save Array"() -> (w1127:string[][])
                n646 = Array Size(array=w1127) -> (size(s)=w1133:i32[])
                n647 = Array Subset(array=w1127, index (row)=0, index (col)=0, length (col)=3) -> (w1129:string[][])  [unwired: 1 in]
                n648 = Index Array(array=w1133, index=0) -> (element=w1135:i32)
                n649 = Reshape Array(w1129, w1135) -> (w1128:string[])
                n650 = Search 1D Array(1D array=w1128, element=w1136) -> (index of element=w1139:i32)  [unwired: 1 in]
                n651 = Equal?(x=w1139, y=-1) -> (x = y?=w1138:bool)
                n652 = case shown="True" w1138 {
                  tunnel: w1127 -> [w1149 w1157]
                  tunnel: w1139 -> [w1146 _]
                  tunnel: [w1145 w1156] -> w1137
                  tunnel: w1128 -> [_ w1155]
                  tunnel: w1136 -> [_ w1154]
                  frame False {
                    # "New Data File"
                    n653 = local read "Calculated Values Cluster"() -> (w1142:T9)
                    n654 = Unbundle By Name(w1142) -> ("Off Current"=w1141:dbl)
                    n655 = Divide(x=w1146, y=3) -> (x/y=w1148:dbl)
                    n656 = Format Value(format string="%#g", value (0)=w1141) -> (output string=w1143:string)  [unwired: 1 in]
                    n657 = To Word Integer(number=w1148) -> (16bit integer=w1147:i16)
                    n658 = Replace Array Subset(array=w1149, new element=w1143, index (row)=w1147, index (col)=1) -> (w1145:string[][])
                  }
                  frame True {
                    # "Old Data File"
                    n659 = local read "Calculated Values Cluster"() -> (w1153:T9)
                    n660 = Unbundle By Name(w1153) -> ("Off Current"=w1152:dbl)
                    n661 = Search 1D Array(1D array=w1155, element="On/Off I-Sat:") -> (index of element=w1162:i32)  [unwired: 1 in]
                    n662 = Divide(x=w1162, y=3) -> (x/y=w1163:dbl)
                    n663 = To Word Integer(number=w1163) -> (16bit integer=w1161:i16)
                    n664 = Format Value(format string="%#g", value (0)=w1152) -> (output string=w1166:string)  [unwired: 1 in]
                    n665 = Build Array(w1154, w1166) -> (w1159:string[])
                    n666 = Increment(x=w1161) -> (x+1=w1160:i16)
                    n667 = Insert Into Array(array=w1157, index (row)=w1160, new element=w1159) -> (w1156:string[][])  [unwired: 1 in]
                  }
                }
                n668 = local write "Save Array"(w1137) -> ()
              }
              frame #9 {
                w1168 = "Vt-Sat (V):"
                n669 = local read "Save Array"() -> (w1169:string[][])
                n670 = Array Size(array=w1169) -> (size(s)=w1174:i32[])
                n671 = Array Subset(array=w1169, index (row)=0, index (col)=0, length (col)=3) -> (w1170:string[][])  [unwired: 1 in]
                n672 = Index Array(array=w1174, index=0) -> (element=w1176:i32)
                n673 = Reshape Array(w1170, w1176) -> (w1167:string[])
                n674 = Search 1D Array(1D array=w1167, element=w1168) -> (index of element=w1179:i32)  [unwired: 1 in]
                n675 = Equal?(x=w1179, y=-1) -> (x = y?=w1178:bool)
                n676 = case shown="True" w1178 {
                  tunnel: w1169 -> [w1188 w1198]
                  tunnel: w1179 -> [w1184 _]
                  tunnel: [w1183 w1197] -> w1177
                  tunnel: w1168 -> [_ w1196]
                  tunnel: w1167 -> [_ w1195]
                  frame False {
                    n677 = local read "Re-Calculated Values Cluster"() -> (w1182:T9)
                    n678 = Unbundle By Name(w1182) -> ("Vt-Sat"=w1181:dbl)
                    n679 = Divide(x=w1184, y=3) -> (x/y=w1187:dbl)
                    n680 = To Word Integer(number=w1187) -> (16bit integer=w1186:i16)
                    n681 = Number To Fractional String(number=w1181) -> (F-format string=w1185:string)  [unwired: 3 in]
                    n682 = Replace Array Subset(array=w1188, new element=w1185, index (row)=w1186, index (col)=1) -> (w1183:string[][])
                  }
                  frame True {
                    n683 = local read "Re-Calculated Values Cluster"() -> (w1192:T9)
                    n684 = Unbundle By Name(w1192) -> ("Vt-Sat"=w1191:dbl)
                    n685 = Search 1D Array(1D array=w1195, element="Threshold V (V):") -> (index of element=w1194:i32)  [unwired: 1 in]
                    n686 = Divide(x=w1194, y=3) -> (x/y=w1201:dbl)
                    n687 = To Word Integer(number=w1201) -> (16bit integer=w1193:i16)
                    n688 = Format Value(format string="%#g", value (0)=w1191) -> (output string=w1204:string)  [unwired: 1 in]
                    n689 = Build Array(w1196, w1204) -> (w1200:string[])
                    n690 = Replace Array Subset(array=w1198, new element=w1200, index (row)=w1193) -> (w1197:string[][])  [unwired: 1 in]
                  }
                }
                n691 = local write "Save Array"(w1177) -> ()
              }
              frame #10 {
                n692 = disable-structure shown="Disabled" {
                  frame Disabled {
                    n693 = local read "Save Array"() -> (w1205:string[][])
                    n694 = Array Size(array=w1205) -> (size(s)=w1211:i32[])
                    n695 = Array Subset(array=w1205, index (row)=0, index (col)=0, length (col)=3) -> (w1207:string[][])  [unwired: 1 in]
                    n696 = Index Array(array=w1211, index=0) -> (element=w1213:i32)
                    n697 = Reshape Array(w1207, w1213) -> (w1206:string[])
                    n698 = Search 1D Array(1D array=w1206, element="VT-Lin (V):") -> (index of element=w1216:i32)  [unwired: 1 in]
                    n699 = Equal?(x=w1216, y=-1) -> (x = y?=w1215:bool)
                    n700 = case shown="False" w1215 {
                      tunnel: w1205 -> [w1225 w1228]
                      tunnel: w1216 -> [w1222 _]
                      tunnel: [w1221 w1228] -> w1214
                      frame False {
                        n701 = Divide(x=w1222, y=3) -> (x/y=w1224:dbl)
                        n702 = To Word Integer(number=w1224) -> (16bit integer=w1223:i16)
                        n703 = Format Value(format string="%#g") -> (output string=w1219:string)  [unwired: 2 in]
                        n704 = Replace Array Subset(array=w1225, new element=w1219, index (row)=w1223, index (col)=1) -> (w1221:string[][])
                      }
                      frame True {
                      }
                    }
                    n705 = local write "Save Array"(w1214) -> ()
                  }
                  frame Enabled {
                  }
                }
              }
              frame #11 {
                w1229 = "STS-Sat (V/decade):"
                n706 = local read "Save Array"() -> (w1231:string[][])
                n707 = Array Size(array=w1231) -> (size(s)=w1236:i32[])
                n708 = Array Subset(array=w1231, index (row)=0, index (col)=0, length (col)=3) -> (w1232:string[][])  [unwired: 1 in]
                n709 = Index Array(array=w1236, index=0) -> (element=w1238:i32)
                n710 = Reshape Array(w1232, w1238) -> (w1230:string[])
                n711 = Search 1D Array(1D array=w1230, element=w1229) -> (index of element=w1241:i32)  [unwired: 1 in]
                n712 = Equal?(x=w1241, y=-1) -> (x = y?=w1240:bool)
                n713 = case shown="True" w1240 {
                  tunnel: w1231 -> [w1251 w1259]
                  tunnel: w1241 -> [w1248 _]
                  tunnel: [w1247 w1260] -> w1239
                  tunnel: w1230 -> [_ w1258]
                  tunnel: w1229 -> [_ w1257]
                  frame False {
                    # "Current Data File"
                    n714 = local read "Re-Calculated Values Cluster"() -> (w1243:T9)
                    n715 = Unbundle By Name(w1243) -> ("STS"=w1244:dbl)
                    n716 = Divide(x=w1248, y=3) -> (x/y=w1250:dbl)
                    n717 = To Word Integer(number=w1250) -> (16bit integer=w1249:i16)
                    n718 = Format Value(format string="%#g", value (0)=w1244) -> (output string=w1245:string)  [unwired: 1 in]
                    n719 = Replace Array Subset(array=w1251, new element=w1245, index (row)=w1249, index (col)=1) -> (w1247:string[][])
                  }
                  frame True {
                    # "Old Data File"
                    n720 = local read "Re-Calculated Values Cluster"() -> (w1254:T9)
                    n721 = Unbundle By Name(w1254) -> ("STS"=w1255:dbl)
                    n722 = Search 1D Array(1D array=w1258, element="S.T.S. (V/decade):") -> (index of element=w1263:i32)  [unwired: 1 in]
                    n723 = Divide(x=w1263, y=3) -> (x/y=w1264:dbl)
                    n724 = To Word Integer(number=w1264) -> (16bit integer=w1256:i16)
                    n725 = Format Value(format string="%#g", value (0)=w1255) -> (output string=w1267:string)  [unwired: 1 in]
                    n726 = Build Array(w1257, w1267) -> (w1262:string[])
                    n727 = Replace Array Subset(array=w1259, new element=w1262, index (row)=w1256) -> (w1260:string[][])  [unwired: 1 in]
                  }
                }
                n728 = local write "Save Array"(w1239) -> ()
              }
              frame #12 {
                w1268 = "Trap Density-VT (Traps/Vcm^2):"
                n729 = local read "Save Array"() -> (w1270:string[][])
                n730 = Array Size(array=w1270) -> (size(s)=w1275:i32[])
                n731 = Array Subset(array=w1270, index (row)=0, index (col)=0, length (col)=3) -> (w1271:string[][])  [unwired: 1 in]
                n732 = Index Array(array=w1275, index=0) -> (element=w1277:i32)
                n733 = Reshape Array(w1271, w1277) -> (w1269:string[])
                n734 = Search 1D Array(1D array=w1269, element=w1268) -> (index of element=w1280:i32)  [unwired: 1 in]
                n735 = Equal?(x=w1280, y=-1) -> (x = y?=w1279:bool)
                n736 = case shown="True" w1279 {
                  tunnel: w1270 -> [w1290 w1297]
                  tunnel: w1280 -> [w1286 _]
                  tunnel: [w1285 w1298] -> w1278
                  tunnel: w1269 -> [_ w1296]
                  tunnel: w1268 -> [_ w1295]
                  frame False {
                    n737 = local read "Re-Calculated Values Cluster"() -> (w1283:T9)
                    n738 = Unbundle By Name(w1283) -> ("Trap Density-VT"=w1282:dbl)
                    n739 = Divide(x=w1286, y=3) -> (x/y=w1289:dbl)
                    n740 = To Word Integer(number=w1289) -> (16bit integer=w1288:i16)
                    n741 = Format Value(format string="%#g", value (0)=w1282) -> (output string=w1287:string)  [unwired: 1 in]
                    n742 = Replace Array Subset(array=w1290, new element=w1287, index (row)=w1288, index (col)=1) -> (w1285:string[][])
                  }
                  frame True {
                    n743 = local read "Re-Calculated Values Cluster"() -> (w1294:T9)
                    n744 = Unbundle By Name(w1294) -> ("Trap Density-VT"=w1293:dbl)
                    n745 = Search 1D Array(1D array=w1296, element="STS-Sat (V/decade):") -> (index of element=w1303:i32)  [unwired: 1 in]
                    n746 = Divide(x=w1303, y=3) -> (x/y=w1302:dbl)
                    n747 = To Word Integer(number=w1302) -> (16bit integer=w1304:i16)
                    n748 = Format Value(format string="%#g", value (0)=w1293) -> (output string=w1299:string)  [unwired: 1 in]
                    n749 = Build Array(w1295, w1299) -> (w1306:string[])
                    n750 = Increment(x=w1304) -> (x+1=w1305:i16)
                    n751 = Insert Into Array(array=w1297, index (row)=w1305, new element=w1306) -> (w1298:string[][])  [unwired: 1 in]
                  }
                }
                n752 = local write "Save Array"(w1278) -> ()
              }
              frame #13 {
                w1308 = "Trap Density-STS (Traps/Vcm^2):"
                n753 = local read "Save Array"() -> (w1310:string[][])
                n754 = Array Size(array=w1310) -> (size(s)=w1315:i32[])
                n755 = Array Subset(array=w1310, index (row)=0, index (col)=0, length (col)=3) -> (w1311:string[][])  [unwired: 1 in]
                n756 = Index Array(array=w1315, index=0) -> (element=w1317:i32)
                n757 = Reshape Array(w1311, w1317) -> (w1309:string[])
                n758 = Search 1D Array(1D array=w1309, element=w1308) -> (index of element=w1320:i32)  [unwired: 1 in]
                n759 = Equal?(x=w1320, y=-1) -> (x = y?=w1319:bool)
                n760 = case shown="True" w1319 {
                  tunnel: w1310 -> [w1330 w1337]
                  tunnel: w1320 -> [w1327 _]
                  tunnel: [w1326 w1338] -> w1318
                  tunnel: w1309 -> [_ w1336]
                  tunnel: w1308 -> [_ w1335]
                  frame False {
                    n761 = local read "Re-Calculated Values Cluster"() -> (w1323:T9)
                    n762 = Unbundle By Name(w1323) -> ("Trap Density-STS"=w1322:dbl)
                    n763 = Divide(x=w1327, y=3) -> (x/y=w1329:dbl)
                    n764 = To Word Integer(number=w1329) -> (16bit integer=w1328:i16)
                    n765 = Format Value(format string="%#g", value (0)=w1322) -> (output string=w1324:string)  [unwired: 1 in]
                    n766 = Replace Array Subset(array=w1330, new element=w1324, index (row)=w1328, index (col)=1) -> (w1326:string[][])
                  }
                  frame True {
                    n767 = local read "Re-Calculated Values Cluster"() -> (w1334:T9)
                    n768 = Unbundle By Name(w1334) -> ("Trap Density-STS"=w1333:dbl)
                    n769 = Search 1D Array(1D array=w1336, element="Trap Density-VT (Traps/Vcm^2):") -> (index of element=w1343:i32)  [unwired: 1 in]
                    n770 = Divide(x=w1343, y=3) -> (x/y=w1344:dbl)
                    n771 = To Word Integer(number=w1344) -> (16bit integer=w1342:i16)
                    n772 = Format Value(format string="%#g", value (0)=w1333) -> (output string=w1347:string)  [unwired: 1 in]
                    n773 = Build Array(w1335, w1347) -> (w1340:string[])
                    n774 = Increment(x=w1342) -> (x+1=w1341:i16)
                    n775 = Insert Into Array(array=w1337, index (row)=w1341, new element=w1340) -> (w1338:string[][])  [unwired: 1 in]
                  }
                }
                n776 = local write "Save Array"(w1318) -> ()
              }
            }
            n777 = local read "New: Temp"() -> (w855:dbl)
            n778 = local read "New: Width"() -> (w856:dbl)
            n779 = local read "New: Length"() -> (w858:dbl)
            n780 = local read "Index"() -> (w857:string)
            n781 = To Single Precision Float(number=w855) -> (single precision float=w872:sgl)
            n782 = Number To Decimal String(number=w872) -> (decimal integer string=w867:string)  [unwired: 1 in]
            n783 = To Single Precision Float(number=w856) -> (single precision float=w871:sgl)
            n784 = To Single Precision Float(number=w858) -> (single precision float=w870:sgl)
            n785 = Strip Path(path=w854) -> (stripped path=w859:path)  [unwired: 1 out]
            n786 = Number To Decimal String(number=w870) -> (decimal integer string=w865:string)  [unwired: 1 in]
            n787 = Number To Decimal String(number=w871) -> (decimal integer string=w864:string)  [unwired: 1 in]
            n788 = Concatenate Strings("_", w867, "K") -> (w869:string)
            n789 = call "Build Text"("Temp"=w869, "Index"=w857, "Length"=w865, "Width"=w864) -> ("Result"=w863:string)  [unwired: 10 in, 1 out]
            n790 = Path To String(path=w859) -> (string=w861:string)
            n791 = Concatenate Strings(w861, "\\", w863) -> (w862:string)
            n792 = String To Path(string=w862) -> (path=w853:path)
          }
          frame #1 {
            n793 = flat-sequence {
              tunnel: w1351 -> [w1353]
              tunnel: w1350 -> [w1352]
              tunnel: [w1352] -> w1349
              tunnel: w1349 -> [w1359]
              tunnel: w1348 -> [w1358]
              frame #0 {
                n794 = Equal?(x=w1353, y=w1352) -> (x = y?=w1354:bool)
                n795 = case shown="False" w1354 {
                  tunnel: w1353 -> [w1357 _]
                  tunnel: w1352 -> [w1356 _]
                  frame False {
                    n796 = Move(source path=w1357, 9:TRUE, 10:w1356) -> ()  [unwired: 2 in, 3 out]
                  }
                  frame True {
                  }
                }
              }
              frame #1 {
                n797 = local write "Transfer File"(w1359) -> ()
                n798 = call-poly <vilib>:"Write To Spreadsheet File.vi"("2D data"=w1358, "file path (dialog if empty)"=w1359) -> ()  [unwired: 6 in, 1 out]
              }
            }
          }
        }
        n799 = Unbundle By Name(w839) -> ("Save Next"=w838:bool)
        n800 = Cluster To Array(cluster=w844) -> (array=w843:bool[])
        n801 = Boolean Array To Number(Boolean array=w843) -> (number=w842:u32)
        n802 = Equal To 0?(x=w842) -> (x = 0?=w841:bool)
        n803 = case shown="True" w841 {
          tunnel: [MegaAwesome_States."Read Data" w851] -> w840
          tunnel: w838 -> [_ w848]
          frame False {
          }
          frame True {
            n804 = Select(t=MegaAwesome_States."No Event", s=w848, f=MegaAwesome_States."Next File") -> (s? t:f=w851:T2)
          }
        }
      }
      frame "Exit" {
        n805 = flat-sequence {
          tunnel: [w1370] -> w1361
          tunnel: [w1370] -> w1360
          frame #0 {
            w1369 = FALSE
            n806 = property on="Next File" class="Bool (strict)"("Value"=w1369) -> (error out=w1364:errorcluster)  [unwired: 2 in, 1 out]
            n807 = property on="Previous File" class="Bool (strict)"(error in=w1364, "Value"=w1369) -> (error out=w1365:errorcluster)  [unwired: 1 in, 1 out]
            n808 = property on="Save" class="Bool (strict)"(error in=w1365, "Value"=w1369) -> (error out=w1366:errorcluster)  [unwired: 1 in, 1 out]
            n809 = property on="Export" class="Bool (strict)"("Value"=w1369) -> ()  [unwired: 2 in, 2 out]
            n810 = property on="Save Next" class="Bool (strict)"(error in=w1366, "Value"=w1369) -> (error out=w1367:errorcluster)  [unwired: 1 in, 1 out]
            n811 = property on="Discard" class="Bool (strict)"(error in=w1367, "Value"=w1369) -> (error out=w1368:errorcluster)  [unwired: 1 in, 1 out]
            n812 = property on="Save Lines" class="Bool (strict)"(error in=w1368, "Value"=w1369) -> ()  [unwired: 1 in, 2 out]
            n813 = property on="Close" class="Bool (strict)"("Value"=w1369) -> ()  [unwired: 2 in, 2 out]
            n814 = property on="Disable Flag" class="Bool (strict)"("Value"=w1369) -> ()  [unwired: 2 in, 2 out]
            n815 = call "IMAQ Dispose"("All Images? (No)"=TRUE) -> ()  [unwired: 5 in, 1 out]
          }
          frame #1 {
            w1370 = MegaAwesome_States."Exit"
          }
        }
      }
      frame "Save Lines" {
        n816 = Build Path(base path=w1372, name or relative path="ROI") -> (appended path=w1375:path)
        n817 = call <vilib>:"Check if File or Folder Exists.vi"("path"=w1375) -> ("file or folder exists?"=w1373:bool, "dup path"=w1376:path)  [unwired: 8 in, 1 out]
        n818 = case shown="False" w1373 {
          tunnel: w1376 -> [w1384 w1385]
          tunnel: [w1383 w1385] -> w1380
          frame False {
            n819 = Create Folder(path (use dialog)=w1384) -> (created path=w1383:path)  [unwired: 2 in, 2 out]
          }
          frame True {
          }
        }
        n820 = local read "Index"() -> (w1371:string)
        n821 = property on="Image Out" class="ImageControl"() -> ("ROI"=w1377:T12)  [unwired: 2 in, 2 out]
        n822 = Build Path(base path=w1380, name or relative path=w1371) -> (appended path=w1379:path)
        n823 = Flatten To String(anything=w1377) -> (data string=w1378:string)  [unwired: 3 in, 2 out]
        n824 = Write to Text File(file (use dialog)=w1379, text=w1378) -> ()  [unwired: 2 in, 3 out]
      }
      frame "Export" {
        n825 = flat-sequence {
          tunnel: ["Independant Variable:"] -> w1386
          tunnel: w1387 -> [w1442]
          tunnel: w1386 -> [w1441]
          frame #0 {
            n826 = stacked-sequence {
              tunnel: "Independant Variable:" -> [w1391 w1396 w1401 w1406 w1411 w1416 w1421 w1426 w1431 w1436]
              frame #0 {
                n827 = Equal?(x=w1391, y="Length (um):") -> (x = y?=w1392:bool)
                n828 = case shown="True" w1392 {
                  frame False {
                  }
                  frame True {
                    n829 = local write "X Axis Display Type"("1") -> ()
                    n830 = local write "Opj X Axis"("2") -> ()
                  }
                }
              }
              frame #1 {
                n831 = Equal?(x=w1396, y="Sample Temp (K):") -> (x = y?=w1397:bool)
                n832 = case shown="True" w1397 {
                  frame False {
                  }
                  frame True {
                    n833 = local write "X Axis Display Type"("1") -> ()
                    n834 = local write "Opj X Axis"("1") -> ()
                  }
                }
              }
              frame #2 {
                n835 = Equal?(x=w1401, y="Mobility-Sat (cm^2/Vs):") -> (x = y?=w1402:bool)
                n836 = case shown="True" w1402 {
                  frame False {
                  }
                  frame True {
                    n837 = local write "X Axis Display Type"("2") -> ()
                    n838 = local write "Opj X Axis"("2") -> ()
                  }
                }
              }
              frame #3 {
                n839 = Equal?(x=w1406, y="Mobility-Lin (cm^2/Vs):") -> (x = y?=w1407:bool)
                n840 = case shown="True" w1407 {
                  frame False {
                  }
                  frame True {
                    n841 = local write "X Axis Display Type"("2") -> ()
                    n842 = local write "Opj X Axis"("2") -> ()
                  }
                }
              }
              frame #4 {
                n843 = Equal?(x=w1411, y="On/Off I-Sat:") -> (x = y?=w1412:bool)
                n844 = case shown="True" w1412 {
                  frame False {
                  }
                  frame True {
                    n845 = local write "X Axis Display Type"("2") -> ()
                    n846 = local write "Opj X Axis"("2") -> ()
                  }
                }
              }
              frame #5 {
                n847 = Equal?(x=w1416, y="Off I-Sat (A):") -> (x = y?=w1417:bool)
                n848 = case shown="True" w1417 {
                  frame False {
                  }
                  frame True {
                    n849 = local write "X Axis Display Type"("2") -> ()
                    n850 = local write "Opj X Axis"("2") -> ()
                  }
                }
              }
              frame #6 {
                n851 = Equal?(x=w1421, y="Vt-Sat (V):") -> (x = y?=w1422:bool)
                n852 = case shown="True" w1422 {
                  frame False {
                  }
                  frame True {
                    n853 = local write "X Axis Display Type"("1") -> ()
                    n854 = local write "Opj X Axis"("1") -> ()
                  }
                }
              }
              frame #7 {
                n855 = Equal?(x=w1426, y="STS-Sat (V/decade):") -> (x = y?=w1427:bool)
                n856 = case shown="True" w1427 {
                  frame False {
                  }
                  frame True {
                    n857 = local write "X Axis Display Type"("1") -> ()
                    n858 = local write "Opj X Axis"("1") -> ()
                  }
                }
              }
              frame #8 {
                n859 = Equal?(x=w1431, y="Trap Density-VT (Traps/Vcm^2):") -> (x = y?=w1432:bool)
                n860 = case shown="True" w1432 {
                  frame False {
                  }
                  frame True {
                    n861 = local write "X Axis Display Type"("2") -> ()
                    n862 = local write "Opj X Axis"("2") -> ()
                  }
                }
              }
              frame #9 {
                n863 = Equal?(x=w1436, y="Trap Density-STS (Traps/Vcm^2):") -> (x = y?=w1437:bool)
                n864 = case shown="True" w1437 {
                  frame False {
                  }
                  frame True {
                    n865 = local write "X Axis Display Type"("2") -> ()
                    n866 = local write "Opj X Axis"("2") -> ()
                  }
                }
              }
            }
          }
          frame #1 {
            n867 = local read "Transfer Folder"() -> (w1446:path)
            n868 = Build Path(base path=w1446, name or relative path="Stats") -> (appended path=w1447:path)
            n869 = call <vilib>:"Check if File or Folder Exists.vi"("path"=w1447) -> ("file or folder exists?"=w1461:bool, "dup path"=w1460:path)  [unwired: 8 in, 1 out]
            n870 = call <userlib>:"OA_ConnectToOrigin.vi"() -> ("error out"=w1458:errorcluster, "Origin.IOApplication"=w1459:refnum<k7>)  [unwired: 8 in]
            n871 = case shown="False" w1461 {
              tunnel: w1460 -> [w1634 w1635]
              tunnel: [w1633 w1635] -> w1445
              frame False {
                n872 = Create Folder(path (use dialog)=w1634) -> (created path=w1633:path)  [unwired: 2 in, 2 out]
              }
              frame True {
              }
            }
            n873 = call "File Dialog"("start path"=w1447) -> ("selected path"=w1449:path)  [unwired: 11 in, 3 out]
            n874 = call <userlib>:"OA_Load.vi"("error in (no error)"=w1458, "Path"=w1442, "Origin.IOApplication"=w1459) -> ("error out"=w1456:errorcluster, "Origin.IOApplication"=w1457:refnum<k7>)  [unwired: 1 out]
            n875 = call "OAExecute.vi"("script"="document -m 3;", "Error IO"=w1456, "Origin.IOApplication"=w1457) -> ("Error IO Out"=w1454:errorcluster, "Origin.IOApplication"=w1455:refnum<k7>)  [unwired: 1 in, 1 out]
            n876 = stacked-sequence {
              tunnel: w1446 -> [w1472 w1502 w1514 w1536 w1556 w1577 w1598 w1621]
              tunnel: w1445 -> [w1473 w1501 w1515 w1535 w1557 w1578 w1599 w1622]
              tunnel: w1455 -> [w1475 w1499 w1517 w1538 w1559 w1580 w1601 w1624]
              tunnel: w1454 -> [w1474 w1500 w1516 w1537 w1558 w1579 w1600 w1623]
              tunnel: [_ _ _ _ _ _ _ w1619] -> w1444
              tunnel: [_ _ _ _ _ _ _ w1620] -> w1443
              tunnel: w1441 -> [w1471 w1492 w1513 w1534 w1555 w1576 w1597 w1618]
              frame #0 {
                n877 = local read "X Axis Display Type"() -> (w1463:string)
                n878 = local read "Opj X Axis"() -> (w1468:string)
                n879 = Concatenate Strings("window -a MOBLGraph;\nlayer.x.type=", w1468, "; layer.x.label.numFormat = ", w1463, "; Y3 = 1; X3 = 1;", "window -a MOBLTable;\nwindow -s TV;") -> (w1466:string)
                n880 = call "Param_Analysis_7_24b_JW.vi"("Independant Variable"=w1471, "error in (no error)"=w1474, "Data Folder"=w1472, "Parameter String"="Mobility-Lin (cm^2/Vs):", "Parameter Name"="Mobility-Lin", "Stats Folder"=w1473) -> ("error out"=w1477:errorcluster, "Output Array"=w1479:string[][], "Variables"=w1470:T27)  [unwired: 2 in, 1 out]
                n881 = call "Origin_Export_7_27a_JW.vi"("Input Conditions"=w1470, "Analysis Array"=w1479, "error in (no error)"=w1477, "Parameter Worksheet Name"="[MOBLTable]Mobilities", "Parameter Folder Script"="pe_cd \"Mobility-Lin\";", "Origin.IOApplication"=w1475) -> ("error out"=w1476:errorcluster, "reference out"=w1478:refnum<k7>)  [unwired: 3 in, 1 out]
                n882 = call "OAExecute.vi"("script"=w1466, "Error IO"=w1476, "Origin.IOApplication"=w1478) -> ()  [unwired: 1 in, 3 out]
              }
              frame #1 {
                n883 = local read "X Axis Display Type"() -> (w1484:string)
                n884 = local read "Opj X Axis"() -> (w1489:string)
                n885 = Concatenate Strings("window -a MOBSGraph;\nlayer.x.type=", w1489, "; layer.x.label.numFormat = ", w1484, "; Y3 = 1; X3 = 1;", "window -a MOBSTable;\nwindow -s TV;") -> (w1487:string)
                n886 = call "Param_Analysis_7_24b_JW.vi"("Independant Variable"=w1492, "error in (no error)"=w1500, "Data Folder"=w1502, "Parameter String"="Mobility-Sat (cm^2/Vs):", "Parameter Name"="Mobility-Sat", "Stats Folder"=w1501) -> ("error out"=w1495:errorcluster, "Output Array"=w1493:string[][], "Variables"=w1491:T27)  [unwired: 2 in, 1 out]
                n887 = call "Origin_Export_7_27a_JW.vi"("Input Conditions"=w1491, "Analysis Array"=w1493, "error in (no error)"=w1495, "Parameter Worksheet Name"="[MOBSTable]Mobilities", "Parameter Folder Script"="pe_cd \"Mobility-Sat\";", "Origin.IOApplication"=w1499) -> ("error out"=w1494:errorcluster, "reference out"=w1496:refnum<k7>)  [unwired: 3 in, 1 out]
                n888 = call "OAExecute.vi"("script"=w1487, "Error IO"=w1494, "Origin.IOApplication"=w1496) -> ()  [unwired: 1 in, 3 out]
              }
              frame #2 {
                n889 = local read "X Axis Display Type"() -> (w1505:string)
                n890 = local read "Opj X Axis"() -> (w1510:string)
                n891 = Concatenate Strings("window -a NSTSGraph;\nlayer.x.type=", w1510, "; layer.x.label.numFormat = ", w1505, "; Y3 = 1; X3 = 1;", "window -a NSTSTable;\nwindow -s TV;") -> (w1508:string)
                n892 = call "Param_Analysis_7_24b_JW.vi"("Independant Variable"=w1513, "error in (no error)"=w1516, "Data Folder"=w1514, "Parameter String"="Trap Density-STS (Traps/Vcm^2):", "Parameter Name"="Trap Density-STS", "Stats Folder"=w1515) -> ("error out"=w1520:errorcluster, "Output Array"=w1518:string[][], "Variables"=w1512:T27)  [unwired: 2 in, 1 out]
                n893 = call "Origin_Export_7_27a_JW.vi"("Input Conditions"=w1512, "Analysis Array"=w1518, "error in (no error)"=w1520, "Parameter Worksheet Name"="[NSTSTable]Trap Densities", "Parameter Folder Script"="pe_cd \"N-STS\";", "Origin.IOApplication"=w1517) -> ("error out"=w1519:errorcluster, "reference out"=w1521:refnum<k7>)  [unwired: 3 in, 1 out]
                n894 = call "OAExecute.vi"("script"=w1508, "Error IO"=w1519, "Origin.IOApplication"=w1521) -> ()  [unwired: 1 in, 3 out]
              }
              frame #3 {
                n895 = local read "X Axis Display Type"() -> (w1526:string)
                n896 = local read "Opj X Axis"() -> (w1531:string)
                n897 = call "Param_Analysis_7_24b_JW.vi"("Independant Variable"=w1534, "error in (no error)"=w1537, "Data Folder"=w1536, "Parameter String"="Trap Density-VT (Traps/Vcm^2):", "Parameter Name"="Trap Density-Vt", "Stats Folder"=w1535) -> ("error out"=w1541:errorcluster, "Output Array"=w1539:string[][], "Variables"=w1533:T27)  [unwired: 2 in, 1 out]
                n898 = Concatenate Strings("window -a NVtGraph;\nlayer.x.type=", w1531, "; layer.x.label.numFormat = ", w1526, "; Y3 = 1; X3 = 1;", "window -a NVtTable;\nwindow -s TV;") -> (w1529:string)
                n899 = call "Origin_Export_7_27a_JW.vi"("Input Conditions"=w1533, "Analysis Array"=w1539, "error in (no error)"=w1541, "Parameter Worksheet Name"="[NVTTable]Trap Densities", "Parameter Folder Script"="pe_cd \"N-Vt\";", "Origin.IOApplication"=w1538) -> ("error out"=w1540:errorcluster, "reference out"=w1542:refnum<k7>)  [unwired: 3 in, 1 out]
                n900 = call "OAExecute.vi"("script"=w1529, "Error IO"=w1540, "Origin.IOApplication"=w1542) -> ()  [unwired: 1 in, 3 out]
              }
              frame #4 {
                n901 = local read "X Axis Display Type"() -> (w1547:string)
                n902 = local read "Opj X Axis"() -> (w1552:string)
                n903 = Concatenate Strings("window -a OffIGraph;\nlayer.x.type=", w1552, "; layer.x.label.numFormat = ", w1547, "; Y3 = 1; X3 = 1;", "window -a OffITable;\nwindow -s TV;") -> (w1550:string)
                n904 = call "Param_Analysis_7_24b_JW.vi"("Independant Variable"=w1555, "error in (no error)"=w1558, "Data Folder"=w1556, "Parameter String"="Off I-Sat (A):", "Parameter Name"="Off I-Sat", "Stats Folder"=w1557) -> ("error out"=w1562:errorcluster, "Output Array"=w1560:string[][], "Variables"=w1554:T27)  [unwired: 2 in, 1 out]
                n905 = call "Origin_Export_7_27a_JW.vi"("Input Conditions"=w1554, "Analysis Array"=w1560, "error in (no error)"=w1562, "Parameter Worksheet Name"="[OffItable]OffCurrents", "Parameter Folder Script"="pe_cd \"OffI-Sat\";", "Origin.IOApplication"=w1559) -> ("error out"=w1561:errorcluster, "reference out"=w1563:refnum<k7>)  [unwired: 3 in, 1 out]
                n906 = call "OAExecute.vi"("script"=w1550, "Error IO"=w1561, "Origin.IOApplication"=w1563) -> ()  [unwired: 1 in, 3 out]
              }
              frame #5 {
                n907 = local read "X Axis Display Type"() -> (w1568:string)
                n908 = local read "Opj X Axis"() -> (w1573:string)
                n909 = Concatenate Strings("window -a OnOffGraph;\nlayer.x.type=", w1573, "; layer.x.label.numFormat = ", w1568, "; Y3 = 1; X3 = 1;", "window -a OnOffTable;\nwindow -s TV;") -> (w1571:string)
                n910 = call "Param_Analysis_7_24b_JW.vi"("Independant Variable"=w1576, "error in (no error)"=w1579, "Data Folder"=w1577, "Parameter String"="On/Off I-Sat:", "Parameter Name"="OnOff Ratio", "Stats Folder"=w1578) -> ("error out"=w1583:errorcluster, "Output Array"=w1581:string[][], "Variables"=w1575:T27)  [unwired: 2 in, 1 out]
                n911 = call "Origin_Export_7_27a_JW.vi"("Input Conditions"=w1575, "Analysis Array"=w1581, "error in (no error)"=w1583, "Parameter Worksheet Name"="[OnOffTable]On/Off Ratios", "Parameter Folder Script"="pe_cd \"OnOff-Ratio\";", "Origin.IOApplication"=w1580) -> ("error out"=w1582:errorcluster, "reference out"=w1584:refnum<k7>)  [unwired: 3 in, 1 out]
                n912 = call "OAExecute.vi"("script"=w1571, "Error IO"=w1582, "Origin.IOApplication"=w1584) -> ()  [unwired: 1 in, 3 out]
              }
              frame #6 {
                n913 = local read "X Axis Display Type"() -> (w1589:string)
                n914 = local read "Opj X Axis"() -> (w1594:string)
                n915 = call "Param_Analysis_7_24b_JW.vi"("Independant Variable"=w1597, "error in (no error)"=w1600, "Data Folder"=w1598, "Parameter String"="STS-Sat (V/decade):", "Parameter Name"="STS-Sat", "Stats Folder"=w1599) -> ("error out"=w1604:errorcluster, "Output Array"=w1602:string[][], "Variables"=w1596:T27)  [unwired: 2 in, 1 out]
                n916 = Concatenate Strings("window -a SGraph;\nlayer.x.type=", w1594, "; layer.x.label.numFormat = ", w1589, "; Y3 = 1; X3 = 1;", "window -a STable;\nwindow -s TV;") -> (w1592:string)
                n917 = call "Origin_Export_7_27a_JW.vi"("Input Conditions"=w1596, "Analysis Array"=w1602, "error in (no error)"=w1604, "Parameter Worksheet Name"="[STable]Threshold Swing", "Parameter Folder Script"="pe_cd \"STS-Sat\";", "Origin.IOApplication"=w1601) -> ("error out"=w1603:errorcluster, "reference out"=w1605:refnum<k7>)  [unwired: 3 in, 1 out]
                n918 = call "OAExecute.vi"("script"=w1592, "Error IO"=w1603, "Origin.IOApplication"=w1605) -> ()  [unwired: 1 in, 3 out]
              }
              frame #7 {
                n919 = local read "X Axis Display Type"() -> (w1610:string)
                n920 = local read "Opj X Axis"() -> (w1615:string)
                n921 = Concatenate Strings("window -a VtGraph;\nlayer.x.type=", w1615, "; layer.x.label.numFormat = ", w1610, "; Y3 = 1; X3 = 1;", "window -a VtTable;\nwindow -s TV;") -> (w1613:string)
                n922 = call "Param_Analysis_7_24b_JW.vi"("Independant Variable"=w1618, "error in (no error)"=w1623, "Data Folder"=w1621, "Parameter String"="Vt-Sat (V):", "Parameter Name"="Vt-Sat", "Stats Folder"=w1622) -> ("error out"=w1627:errorcluster, "Output Array"=w1625:string[][], "Variables"=w1617:T27)  [unwired: 2 in, 1 out]
                n923 = call "Origin_Export_7_27a_JW.vi"("Input Conditions"=w1617, "Analysis Array"=w1625, "error in (no error)"=w1627, "Parameter Worksheet Name"="[VtTable]Threshold Voltages", "Parameter Folder Script"="pe_cd \"Vt-Sat\";", "Origin.IOApplication"=w1624) -> ("error out"=w1626:errorcluster, "reference out"=w1628:refnum<k7>)  [unwired: 3 in, 1 out]
                n924 = call "OAExecute.vi"("script"=w1613, "Error IO"=w1626, "Origin.IOApplication"=w1628) -> ("Error IO Out"=w1619:errorcluster, "Origin.IOApplication"=w1620:refnum<k7>)  [unwired: 1 in, 1 out]
              }
            }
            n925 = Path To String(path=w1449) -> (string=w1448:string)
            n926 = call "OAExecute.vi"("script"="pe_cd /; ", "Error IO"=w1444, "Origin.IOApplication"=w1443) -> ("Error IO Out"=w1450:errorcluster, "Origin.IOApplication"=w1451:refnum<k7>)  [unwired: 1 in, 1 out]
            n927 = call <userlib>:"OASaveProject.vi"("path"=w1448, "Error IO"=w1450, "Origin.IOApplication"=w1451) -> ()  [unwired: 3 out]
          }
        }
      }
    }
    "Current State" <- w15
    "Folder Index" <- w27
    n928 = Wait (ms)(milliseconds to wait=w21) -> ()  [unwired: 1 out]
    n929 = Equal?(x=w12, y=MegaAwesome_States."Exit") -> (x = y?=w14:bool)
  }
  n930 = call "Close LabView?"("Enable"=w2) -> ("OK"=w1:bool)  [unwired: 17 in, 1 out]
  n931 = Quit LabVIEW(quit? (T)=w1) -> ()
